vi "Strategy 5_Autotuning PID_With GUI_Modified for Testing - Backup.vi"() -> ()   [LabVIEW 2018]
doc: "This example demonstrates how to use the PID Design function to obtain PID parameters based on measured process."
uses:
  <vilib>/DAQmx/write.llb/DAQmx Write (Digital 1D Bool 1Chan 1Samp).vi
  <vilib>/DAQmx/read.llb/DAQmx Read (Analog 1D DBL NChan 1Samp).vi
  <vilib>/Instr/_visa.llb/VISA Configure Serial Port (Instr).vi
  <vilib>/DAQmx/create/channels.llb/DAQmx Create Channel (DO-Digital Output).vi
  <vilib>/DAQmx/miscellaneous.llb/DAQmx Fill In Error Info.vi
  <vilib>/addons/control/pid/pid.llb/PID Advanced (DBL).vi
  <vilib>/addons/control/pid/autopid.llb/PID Autotuning Design (Ziegler-Nichols).vi
  <vilib>/addons/control/pid/autopid.llb/PID Autotuning Design (Cohen-Coon).vi
  <vilib>/addons/control/pid/autopid.llb/PID Autotuning Design (Chien-Hrones-Reswick).vi
  <vilib>/addons/control/pid/autopid.llb/PID Autotuning Design (Internal Model Control).vi
  <vilib>/addons/control/pid/NI_PID_autopid.lvlib
  <vilib>/addons/control/pid/NI_PID_pid.lvlib
  <vilib>/ptbypt/NI_PtbyPt.lvlib
panel:
  in  "Set Point 1,5":dbl
  out "Real time Data 1,5":dbl[][](graph)
  in  "Set Point 3,4":dbl
  out "Real time Data 3,4":dbl[][](graph)
  in  "Set Point 2":dbl
  out "Real time Data 2":dbl[][](graph)
  in  "Set Point 7":dbl
  out "Real time Data 7":dbl[][](graph)
  in  "Set Point  6,8,9,10":dbl
  out "Real time Data 6,8,9,10":dbl[][](graph)
  in  "Set Point 11,12":dbl
  out "Real time Data -11,12":dbl[][](graph)
  out "error out":errorcluster {"code" format="%.0x"}
  in  "XYZAER":T1(array[cluster]) {"r" format="%1_6f"; "e" format="%1_6f"; "a" format="%1_6f"; "z" format="%1_6f"; "y" format="%1_6f"; "x" format="%1_6f"}
  out "Start Time Text":string
  out "Stop Time Text":string
  out "Elapsed Time Text":string
  out "HostFrameCount":u32
  out "Loop Iter":i32
  out "PnoData":bool
  in  "stop":bool
  out "?":bool
  in  "Muscle Control":T2(tab)=enum."M-11,12"
  out "Tuned PID gains 12":T3={"proportional gain (Kc)"=1.9838195929127882, "integral time (Ti, min)"=0.01995856284686879, "derivative time (Td, min)"=0.0} {"derivative time (Td, min)" format="%#.6g"; "integral time (Ti, min)" format="%#.6g"; "proportional gain (Kc)" format="%#.6g"}
  in  "Accept gain 12":bool
  in  "Control 12":T4(tab)
  in  "Ziegler-Nichols speed 12":u16(ring) items=["Fast", "Normal", "Slow"]
  in  "Tuning specifications 12":u16(ring) items=["Regulator - 0 %", "Regulator -  20%", "Servo - 0%", "Servo - 20%"]
  in  "Multiplicative factor 12":dbl(slide)=1.0 scale=0.01..100.0
  in  "Type of controller 12":u16(ring)=2 items=["P", "PI", "PID"]
  in  "Stop 12":bool
  in  "PID Gains 12":T3={"proportional gain (Kc)"=0.1625, "integral time (Ti, min)"=1.25, "derivative time (Td, min)"=0.0} {"derivative time (Td, min)" format="%#.6g"; "integral time (Ti, min)" format="%#.6g"; "proportional gain (Kc)" format="%#.6g"}
  in  "Autotune 12":bool
  in  "Reinitialize 12":bool
  in  "Excitation 12":dbl=0.5 format="%.2f"
  in  "Automatic 12":bool=TRUE
  in  "MV: 12":dbl(slide)=20.39115328927357 scale=-100.0..100.0
  out "PWM Output 12":bool
  in  "Median sample length 21":i32=100
  in  "INLET 1,5 ON/OFF 3":bool=TRUE
  out "Tuned PID gains 9":T3={"proportional gain (Kc)"=1.9838195929127882, "integral time (Ti, min)"=0.01995856284686879, "derivative time (Td, min)"=0.0} {"derivative time (Td, min)" format="%#.6g"; "integral time (Ti, min)" format="%#.6g"; "proportional gain (Kc)" format="%#.6g"}
  in  "Accept gain 9":bool
  in  "Type of controller 9":u16(ring)=2 items=["P", "PI", "PID"]
  in  "Excitation 9":dbl=0.5 format="%.2f"
  in  "Control 9":T4(tab)
  in  "Ziegler-Nichols speed 9":u16(ring) items=["Fast", "Normal", "Slow"]
  in  "Tuning specifications 9":u16(ring) items=["Regulator - 0 %", "Regulator -  20%", "Servo - 0%", "Servo - 20%"]
  in  "Multiplicative factor 9":dbl(slide)=1.0 scale=0.01..100.0
  in  "Stop 9":bool
  in  "PID Gains 9":T3={"proportional gain (Kc)"=0.1625, "integral time (Ti, min)"=1.25, "derivative time (Td, min)"=0.0} {"derivative time (Td, min)" format="%#.6g"; "integral time (Ti, min)" format="%#.6g"; "proportional gain (Kc)" format="%#.6g"}
  in  "Autotune 9":bool
  in  "Reinitialize 9":bool
  in  "Automatic 9":bool=TRUE
  in  "MV: 9":dbl(slide)=20.39115328927357 scale=-100.0..100.0
  out "PWM Output 9":bool
  in  "Median sample length 18":i32=100
  in  "INLET 3,4 ON/OFF 2":bool=TRUE
  out "Tuned PID gains 8":T3={"proportional gain (Kc)"=1.9838195929127882, "integral time (Ti, min)"=0.01995856284686879, "derivative time (Td, min)"=0.0} {"derivative time (Td, min)" format="%#.6g"; "integral time (Ti, min)" format="%#.6g"; "proportional gain (Kc)" format="%#.6g"}
  in  "Accept gain 8":bool
  in  "Control 8":T4(tab)
  in  "Ziegler-Nichols speed 8":u16(ring) items=["Fast", "Normal", "Slow"]
  in  "Tuning specifications 8":u16(ring) items=["Regulator - 0 %", "Regulator -  20%", "Servo - 0%", "Servo - 20%"]
  in  "Multiplicative factor 8":dbl(slide)=1.0 scale=0.01..100.0
  in  "Type of controller 8":u16(ring)=2 items=["P", "PI", "PID"]
  in  "Stop 8":bool
  in  "PID Gains 8":T3={"proportional gain (Kc)"=0.1625, "integral time (Ti, min)"=1.25, "derivative time (Td, min)"=0.0} {"derivative time (Td, min)" format="%#.6g"; "integral time (Ti, min)" format="%#.6g"; "proportional gain (Kc)" format="%#.6g"}
  in  "Autotune 8":bool
  in  "Reinitialize 8":bool
  in  "Excitation 8":dbl=0.5 format="%.2f"
  in  "Automatic 8":bool=TRUE
  in  "MV: 8":dbl(slide)=20.39115328927357 scale=-100.0..100.0
  out "PWM Output 8":bool
  in  "Median sample length 17":i32=100
  in  "INLET 2 ON/OFF 2":bool=TRUE
  out "Tuned PID gains 7":T3={"proportional gain (Kc)"=1.9838195929127882, "integral time (Ti, min)"=0.01995856284686879, "derivative time (Td, min)"=0.0} {"derivative time (Td, min)" format="%#.6g"; "integral time (Ti, min)" format="%#.6g"; "proportional gain (Kc)" format="%#.6g"}
  in  "Accept gain 7":bool
  in  "Control 7":T4(tab)
  in  "Ziegler-Nichols speed 7":u16(ring) items=["Fast", "Normal", "Slow"]
  in  "Tuning specifications 7":u16(ring) items=["Regulator - 0 %", "Regulator -  20%", "Servo - 0%", "Servo - 20%"]
  in  "Multiplicative factor 7":dbl(slide)=1.0 scale=0.01..100.0
  in  "Type of controller 7":u16(ring)=2 items=["P", "PI", "PID"]
  in  "Stop 7":bool
  in  "PID Gains 7":T3={"proportional gain (Kc)"=0.1625, "integral time (Ti, min)"=1.25, "derivative time (Td, min)"=0.0} {"derivative time (Td, min)" format="%#.6g"; "integral time (Ti, min)" format="%#.6g"; "proportional gain (Kc)" format="%#.6g"}
  in  "Autotune 7":bool
  in  "Reinitialize 7":bool
  in  "Excitation 7":dbl=0.5 format="%.2f"
  in  "Automatic 7":bool=TRUE
  in  "MV: 7":dbl(slide)=20.39115328927357 scale=-100.0..100.0
  out "PWM Output 7":bool
  in  "Median sample length 16":i32=100
  in  "INLET 7 ON/OFF 2":bool=TRUE
  out "Tuned PID gains 6":T3={"proportional gain (Kc)"=1.9838195929127882, "integral time (Ti, min)"=0.01995856284686879, "derivative time (Td, min)"=0.0} {"derivative time (Td, min)" format="%#.6g"; "integral time (Ti, min)" format="%#.6g"; "proportional gain (Kc)" format="%#.6g"}
  in  "Accept gain 6":bool
  in  "Control 6":T4(tab)
  in  "Ziegler-Nichols speed 6":u16(ring) items=["Fast", "Normal", "Slow"]
  in  "Tuning specifications 6":u16(ring) items=["Regulator - 0 %", "Regulator -  20%", "Servo - 0%", "Servo - 20%"]
  in  "Multiplicative factor 6":dbl(slide)=1.0 scale=0.01..100.0
  in  "Type of controller 6":u16(ring)=2 items=["P", "PI", "PID"]
  in  "Stop 6":bool
  in  "PID Gains 6":T3={"proportional gain (Kc)"=0.1625, "integral time (Ti, min)"=1.25, "derivative time (Td, min)"=0.0} {"derivative time (Td, min)" format="%#.6g"; "integral time (Ti, min)" format="%#.6g"; "proportional gain (Kc)" format="%#.6g"}
  in  "Autotune 6":bool
  in  "Reinitialize 6":bool
  in  "Excitation 6":dbl=0.5 format="%.2f"
  in  "Automatic 6":bool=TRUE
  in  "MV: 6":dbl(slide)=20.39115328927357 scale=-100.0..100.0
  out "PWM Output 6":bool
  in  "Median sample length 15":i32=100
  in  "INLET 6 ON/OFF 2":bool=TRUE
  in  "INLET":bool=TRUE
  out "PWM Output":bool
  in  "MV:":dbl(slide)=20.39115328927357 scale=-100.0..100.0
  in  "Median sample length":i32=100
  in  "Excitation":dbl=0.5 format="%.2f"
  in  "Type of controller":u16(ring)=2 items=["P", "PI", "PID"]
  in  "Control":T4(tab)
  in  "Ziegler-Nichols speed":u16(ring) items=["Fast", "Normal", "Slow"]
  in  "Tuning specifications":u16(ring) items=["Regulator - 0 %", "Regulator -  20%", "Servo - 0%", "Servo - 20%"]
  in  "Multiplicative factor":dbl(slide)=1.0 scale=0.01..100.0
  in  "Automatic":bool=TRUE
  in  "Reinitialize":bool
  in  "Accept gain":bool
  out "Tuned PID gains":T3={"proportional gain (Kc)"=1.9838195929127882, "integral time (Ti, min)"=0.01995856284686879, "derivative time (Td, min)"=0.0} {"derivative time (Td, min)" format="%#.6g"; "integral time (Ti, min)" format="%#.6g"; "proportional gain (Kc)" format="%#.6g"}
  in  "Autotune":bool
  in  "PID Gains":T3={"proportional gain (Kc)"=0.1625, "integral time (Ti, min)"=1.25, "derivative time (Td, min)"=0.0} {"derivative time (Td, min)" format="%#.6g"; "integral time (Ti, min)" format="%#.6g"; "proportional gain (Kc)" format="%#.6g"}
  in  "Stop":bool
  in  "M-11,12":i32=5
  in  "M-6,8,9,10":i32=5
  in  "M-7":i32=5
  in  "M-2":i32=5
  in  "M-3,4":i32=5
  in  "M-1,5":i32=5
  out "Stimulus operating point 12":dbl=20.314221540357543
  out "Response operating point 12":dbl=51.08345461694337
  out "Identified Plant Parameters 12":T5={"Plant Gain (K)"=1.7609511324977591, "Time Constant (T)"=1.9621978490901302, "Dead Time (L)"=0.22467425343567116}
  out "Control Output 12":dbl[](graph)
  out "Measurement 12":dbl[](graph)
  out "Stimulus operating point 9":dbl=20.314221540357543
  out "Response operating point 9":dbl=51.08345461694337
  out "Identified Plant Parameters 9":T5={"Plant Gain (K)"=1.7609511324977591, "Time Constant (T)"=1.9621978490901302, "Dead Time (L)"=0.22467425343567116}
  out "Control Output 9":dbl[](graph)
  out "Measurement 9":dbl[](graph)
  out "Identified Plant Parameters":T5={"Plant Gain (K)"=1.7609511324977591, "Time Constant (T)"=1.9621978490901302, "Dead Time (L)"=0.22467425343567116}
  out "Control Output":dbl[](graph)
  out "Measurement":dbl[](graph)
  out "Stimulus operating point":dbl=20.314221540357543
  out "Response operating point":dbl=51.08345461694337
  out "Stimulus operating point 6":dbl=20.314221540357543
  out "Response operating point 6":dbl=51.08345461694337
  out "Identified Plant Parameters 6":T5={"Plant Gain (K)"=1.7609511324977591, "Time Constant (T)"=1.9621978490901302, "Dead Time (L)"=0.22467425343567116}
  out "Control Output 6":dbl[](graph)
  out "Measurement 6":dbl[](graph)
  out "Stimulus operating point 7":dbl=20.314221540357543
  out "Response operating point 7":dbl=51.08345461694337
  out "Identified Plant Parameters 7":T5={"Plant Gain (K)"=1.7609511324977591, "Time Constant (T)"=1.9621978490901302, "Dead Time (L)"=0.22467425343567116}
  out "Control Output 7":dbl[](graph)
  out "Measurement 7":dbl[](graph)
  out "Stimulus operating point 8":dbl=20.314221540357543
  out "Response operating point 8":dbl=51.08345461694337
  out "Identified Plant Parameters 8":T5={"Plant Gain (K)"=1.7609511324977591, "Time Constant (T)"=1.9621978490901302, "Dead Time (L)"=0.22467425343567116}
  out "Control Output 8":dbl[](graph)
  out "Measurement 8":dbl[](graph)
  out "Connected":bool
  out "Running":bool
  out "Position Sensor Data":cluster{dbl, "x":sgl}[](graph)
  out "Sensor Raw Value 2":i32
  in  "COM Port-Sensor 2":refnum<visa-resource-name>="COM5"
  in  "upper/lower infle":enum32{"Page 1", "Page 2"}(tab)
  out "Force in Kilograms":dbl(graph)
  out "Force in Newtons":dbl(graph)
  in  "lower/upper infle":enum32{"Page 1", "Page 2"}(tab)
  out "Force in Newtons 2":dbl(graph)
  out "Force in Kilograms 2":dbl(graph)
  in  "COM Port-Sensor 1":refnum<visa-resource-name>="COM4"
  out "Sensor Raw Value":i32
  in  "Tab Control":T6(tab)
  in  "Instructions":string="Overview: This example demonstrates how to use the PID Autotuning Design to obtain PID parameters based on setpoint and process variable collected in another loop.\nInstructions:\n1. Run the VI and wait until the process variable (PV) reaches near setpoint (SP).\n2.  In the PID Autotuning Design section, select the type of algorithm, type of controller and excitation amplitude for the 'open loop step response'. Then, click Autotune to start the process. Select the Identified Plant Parameter tab and see the results from the identification.\n3.  When the tuned PID gains do not change anymore, the identification is done and you have the option to accept by clicking Accept gain, which will transfer the new gain to PID Gains.\n4. Click the Autotune button again to go back to the automatic control state. You can try different options and repeat this process.\n5. Click Stop to stop the VI.\n"
  # "Pressure Alarm"
  # "Force Sensor Data"
  # "Position Sensor Data"
  # "PID Controller"
  # "PID Autotuning Design"
  # "No additional parameters"
  # "PID Controller"
  # "PID Autotuning Design"
  # "No additional parameters"
  # "PID Controller"
  # "PID Autotuning Design"
  # "No additional parameters"
  # "PID Controller"
  # "PID Autotuning Design"
  # "No additional parameters"
  # "PID Controller"
  # "PID Autotuning Design"
  # "No additional parameters"
  # "Muscle Control"
  # "PID Controller"
  # "PID Autotuning Design"
  # "No additional parameters"
  # "Pressure Cut Off to trigger the alarm"
  # "M-11,12"
  # "M-3,4"
  # "M-1,5"
  # "M-6,8,9,10"
  # "M-7"
  # "M-2"
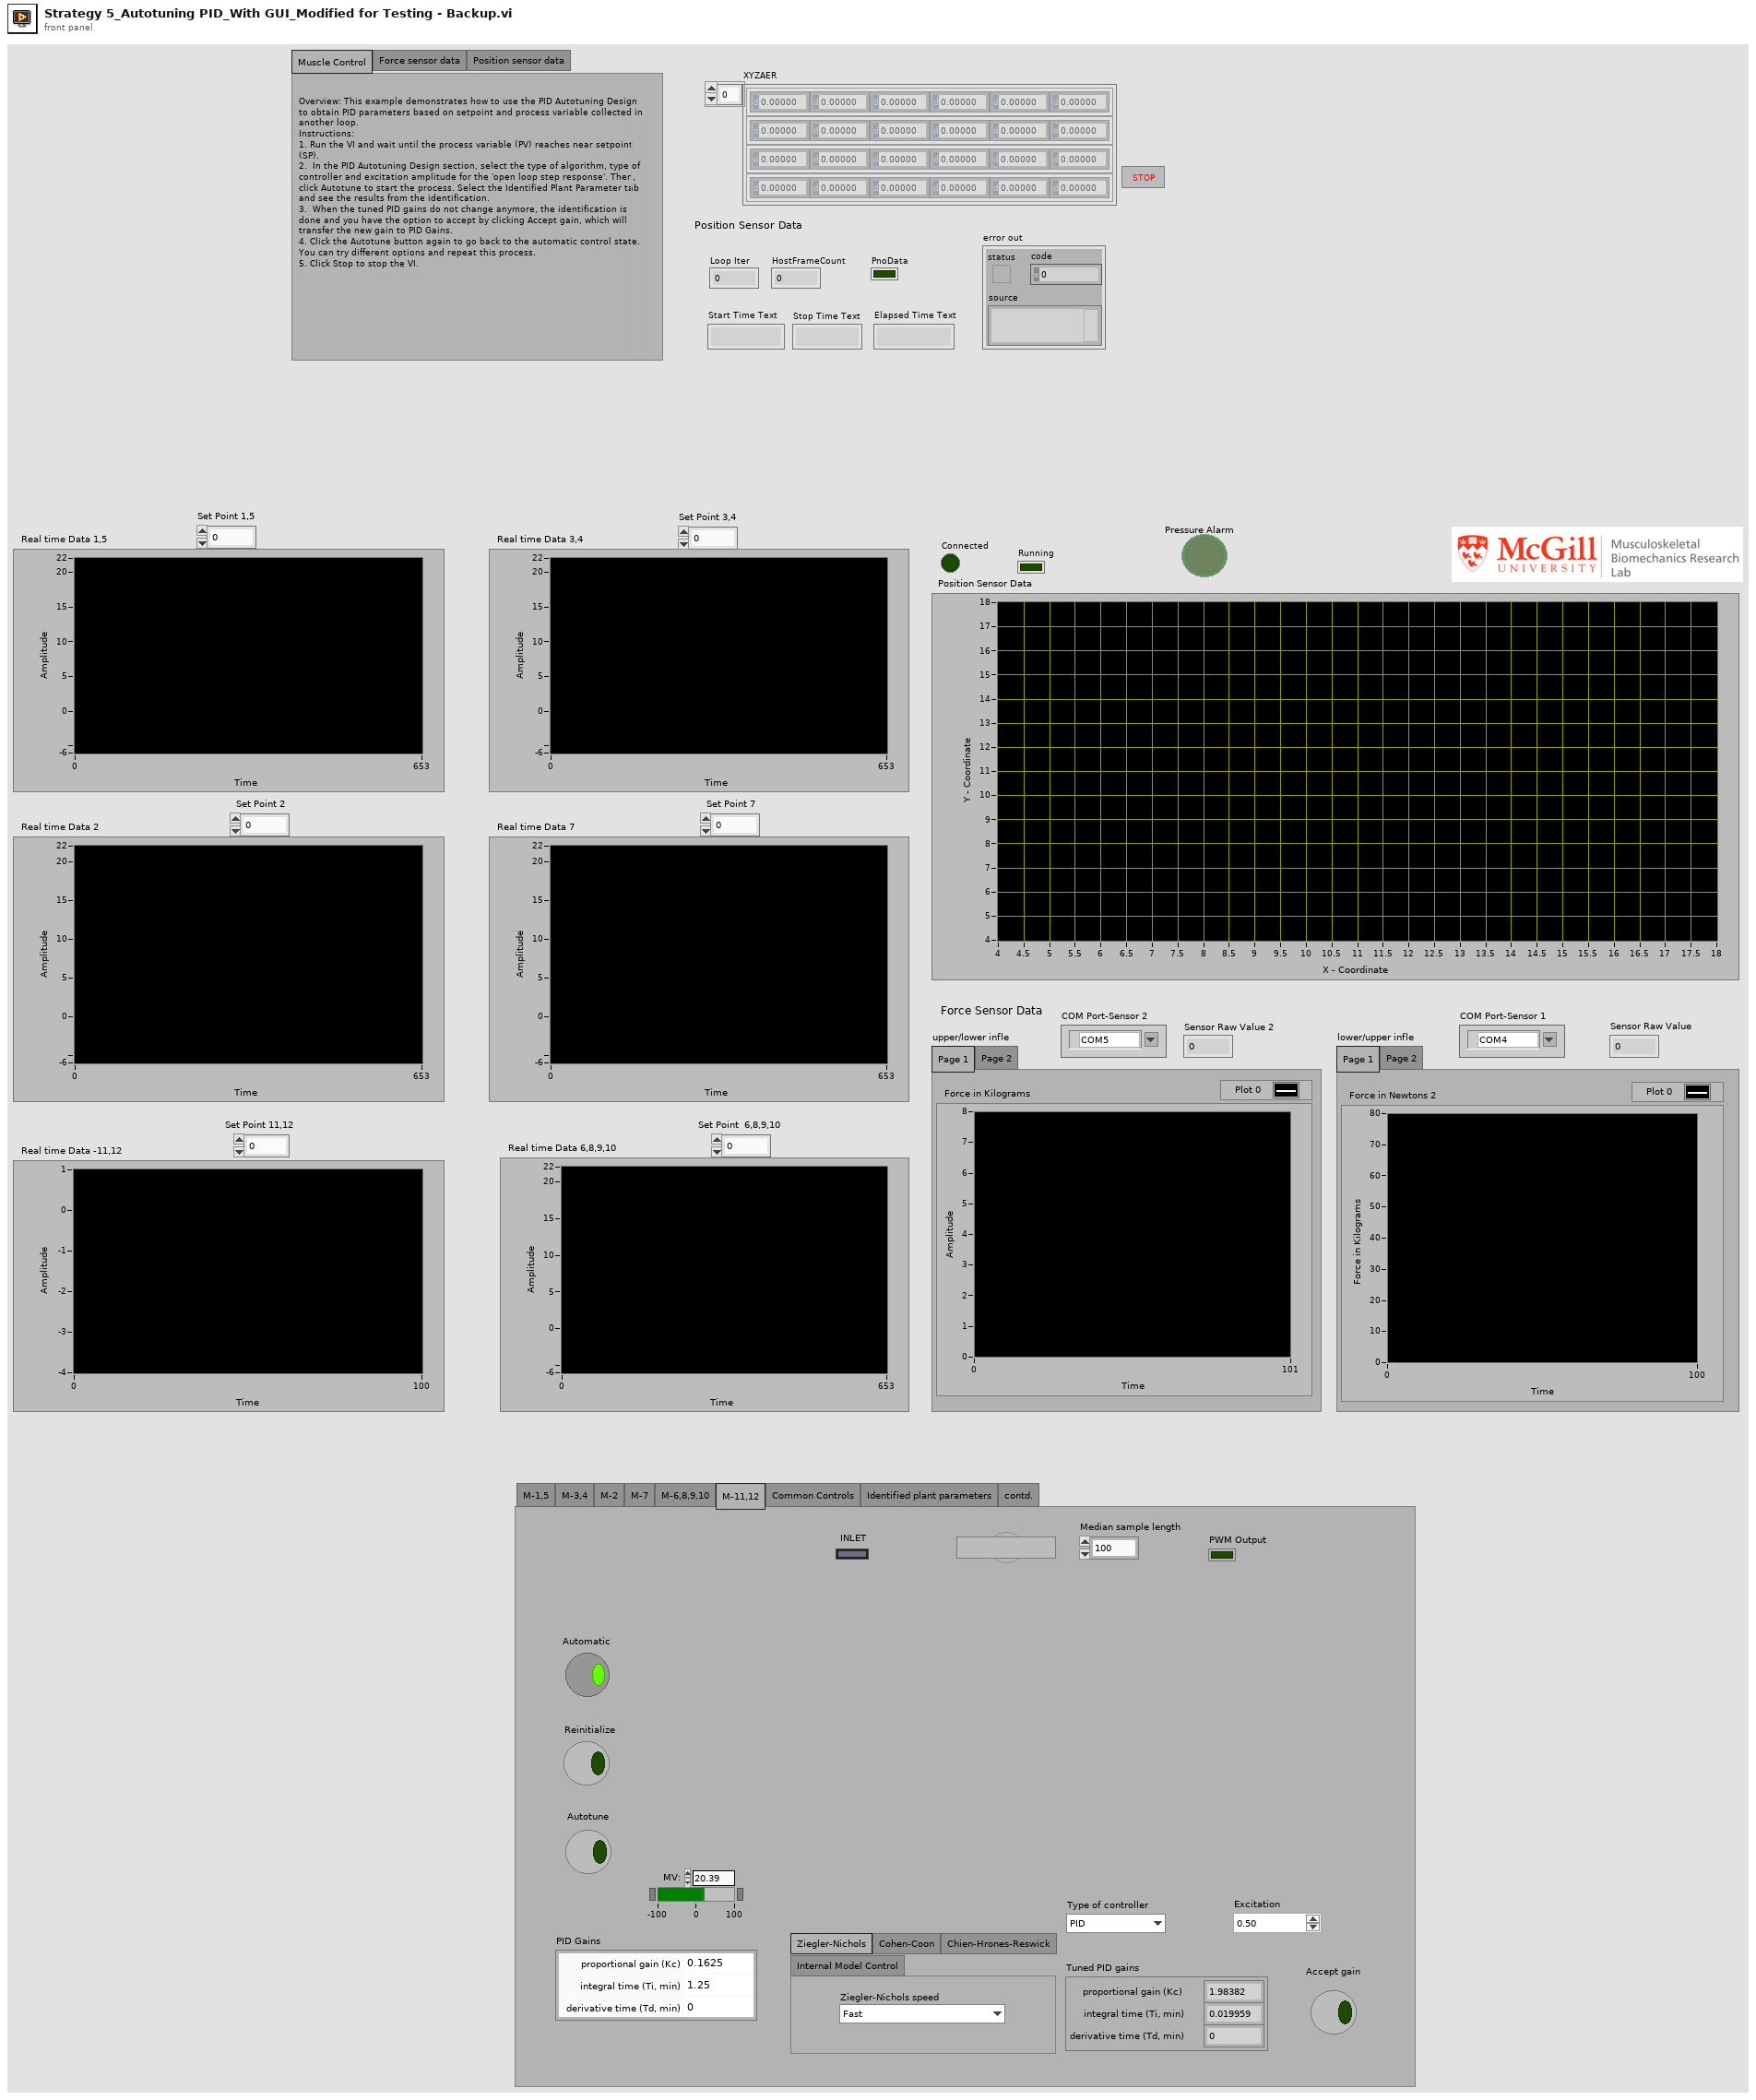
[diagram p1: front panel]
types:
  T1 = cluster{"x":sgl, "y":sgl, "z":sgl, "a":sgl, "e":sgl, "r":sgl}[]
  T2 = enum32{"M-1,5", "M-3,4", "M-2", "M-7", "M-6,8,9,10", "M-11,12", "Common Controls", "Identified plant parameters", "contd."}
  T3 = cluster{"proportional gain (Kc)":dbl, "integral time (Ti, min)":dbl, "derivative time (Td, min)":dbl}
  T4 = enum32{"Ziegler-Nichols", "Cohen-Coon", "Chien-Hrones-Reswick", "Internal Model Control"}
  T5 = cluster{"Plant Gain (K)":dbl, "Time Constant (T)":dbl, "Dead Time (L)":dbl}
  T6 = enum32{"Muscle Control", "Force sensor data", "Position sensor data"}
  T7 = cluster{"static gain":dbl, "lag (s)":dbl, "deadtime (s)":dbl, "load":dbl, "deadband":dbl, "sensor noise":dbl, "initial PV":dbl, "plant noise":dbl}
  T8 = cluster{"x":sgl, "y":sgl, "z":sgl, "a":sgl, "e":sgl, "r":sgl}
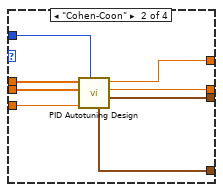
[diagram p2: hidden frame]
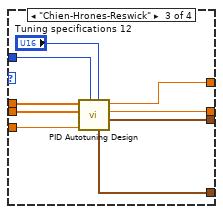
[diagram p3: hidden frame]
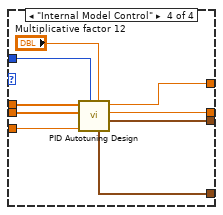
[diagram p4: hidden frame]
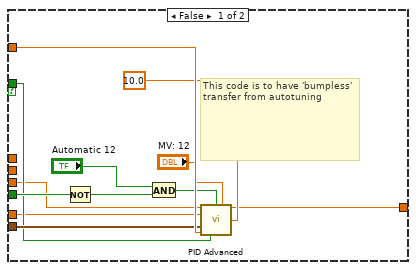
[diagram p6: hidden frame]
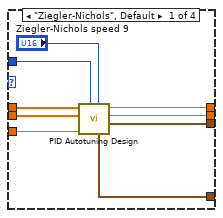
[diagram p7: hidden frame]
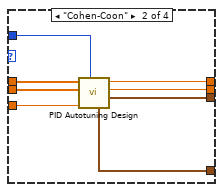
[diagram p8: hidden frame]
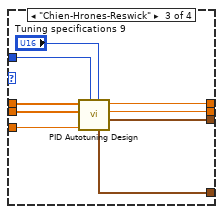
[diagram p9: hidden frame]
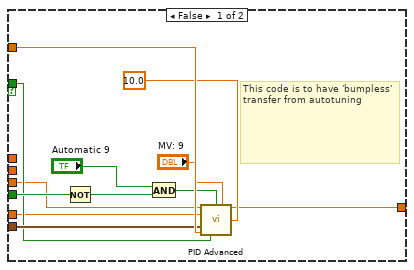
[diagram p11: hidden frame]
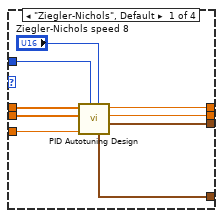
[diagram p12: hidden frame]
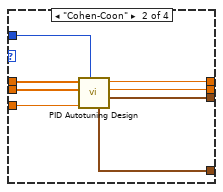
[diagram p13: hidden frame]
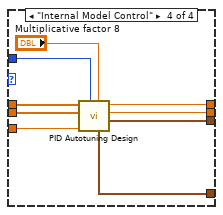
[diagram p14: hidden frame]
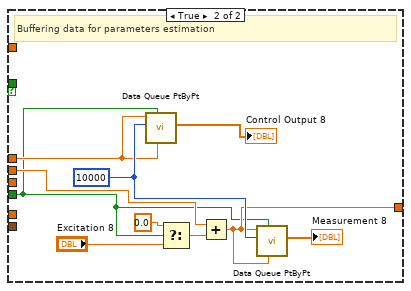
[diagram p16: hidden frame]
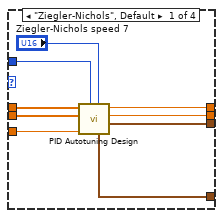
[diagram p17: hidden frame]
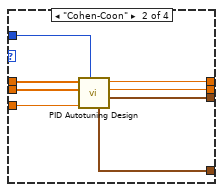
[diagram p18: hidden frame]
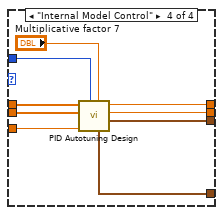
[diagram p19: hidden frame]
diagram:
  w19 = 0.0 ("output")
  w22 = FALSE ("Stop")
  w25 = 0.0 ("output")
  w28 = FALSE ("Stop")
  w31 = 0.0 ("output")
  w34 = FALSE ("Stop")
  w37 = 0.0 ("output")
  w40 = FALSE ("Stop")
  w43 = 0.0 ("output")
  w46 = FALSE ("Stop")
  w51 = 2400  # BufferFrameCount
  w85 = 0.0 ("output")
  w88 = FALSE ("Stop")
  # "Muscle-1,5 PID CONTROL LOOP (Auto Tuning)"
  # "Muscle-3,4 PID CONTROL LOOP (Auto Tuning)"
  # "Muscle-2 PID CONTROL LOOP (Auto Tuning)"
  # "Muscle-7 PID CONTROL LOOP (Auto Tuning)"
  # "Muscle-6,8,9,10 PID CONTROL LOOP (Auto Tuning)"
  # "Muscle-11,12 PID CONTROL LOOP (Auto Tuning)"
  # "FORCE SENSOR CONTROL LOOP"
  # "POSITION SENSOR CONTROL LOOP"
  # "Pressure Alarm"
  # "8. Close Tracker connection."
  # "3. Query Max num sensors supported by the tracker."
  # "4. Allocate raw buffer to hold 2400 frames of data."
  # "5. Start Continuous mode."
  # "7. Stop Continuous mode."
  # "6. Start the loop. Loop exits when Stop Button is hit."
  n1 = Obtain Queue(element data type=0.0) -> (queue out=w12:refnum<queue>)  [unwired: 4 in, 2 out]
  n2 = while {
    shift-left: 0.0 ("Plant Output") -> [w204]
    shift-right: [w199] -> _
    tunnel: w46 -> [_]
    shift-right: [w185] -> _
    shift-left: 0.01 -> [w183]
    shift-right: [w158] -> _
    shift-left: TRUE -> [w182]
    shift-right: [w160] -> _
    shift-left: w43 -> [w181]
    shift-right: [w184] -> _
    shift-left: w43 -> [w180]
    tunnel: [w155] -> w42
    tunnel: [w142] -> w2
    tunnel: w12 -> [w140]
    stop <- "Stop 6" stop-if-true
    w93 = 1 items=["one channel for each line", "one channel for all lines"] ("line grouping")
    w101 = 1 items=["one channel for each line", "one channel for all lines"] ("line grouping")
    w109 = 1 items=["one channel for each line", "one channel for all lines"] ("line grouping")
    w117 = 1 items=["one channel for each line", "one channel for all lines"] ("line grouping")
    w125 = 1 items=["one channel for each line", "one channel for all lines"] ("line grouping")
    w133 = 1 items=["one channel for each line", "one channel for all lines"] ("line grouping")
    w146 = 1 items=["one channel for each line", "one channel for all lines"] ("line grouping")
    w155 = 0.05 ("Sampling Time dt (s)")
    w163 = 1 items=["one channel for each line", "one channel for all lines"] ("line grouping")
    w171 = 0.5 ("x")
    w198 = T7 {"static gain"=2.5, "lag (s)"=2.5, "deadtime (s)"=0.01, "load"=0.0, "deadband"=0.0, "sensor noise"=0.0, "initial PV"=30.0, "plant noise"=0.0}  # Process parameters
    w200 = FALSE  # Integrator ?
    # "Inlet 11"
    # "Exhaust 10"
    # "Inlet 11"
    # "Exhaust 9"
    # "Inlet 11"
    # "Exhaust 8"
    # "C."
    # "Inlet 11"
    # "Exhaust 6"
    # "B."
    # "A."
    # "A.Output to PWM Logic \nB. Simulated Plant\nC. Draw Chart"
    # "Main PID Loop Control"
    n3 = Dequeue Element(queue=w140) -> (element=w141:dbl)  [unwired: 2 in, 3 out]
    n4 = Multiply(x=w155, y=1000.0) -> (x*y=w197:dbl)
    n5 = Not(x="Autotune 6") -> (.not. x?=w201:bool)
    n6 = feedback #1() -> (w206:bool)  [unwired: 1 in]
    n7 = feedback-in #1("Autotune 6") -> ()
    n8 = Wait Until Next ms Multiple(millisecond multiple=w197) -> ()  [unwired: 1 out]
    n9 = Exclusive Or(1:w206, 2:"Autotune 6") -> (0:w205:bool)
    n10 = feedback #2() -> (w203:dbl)  [unwired: 1 in]
    n11 = Multiply(x=w141, y=-1000.0) -> (x*y=w187:dbl)
    n12 = call <vilib>:"Median PtByPt.vi"("sample length"="Median sample length 15", "x"=w187) -> ("median"=w186:dbl)  [unwired: 2 in, 1 out]
    n13 = Square(x=w186) -> (x^2=w194:dbl)
    n14 = Multiply(x=w186, y=16.572) -> (x*y=w190:dbl)
    n15 = Multiply(x=w194, y=-0.06) -> (x*y=w191:dbl)
    n16 = Add(x=w190, y=w191) -> (x+y=w189:dbl)
    n17 = Add(x=-1011.3, y=w189) -> (x+y=w153:dbl)
    n18 = case shown="False" "Autotune 6" {
      tunnel: w155 -> [w221 _]
      tunnel: [w210 w226] -> w160
      tunnel: w204 -> [_ w225]
      tunnel: "PID Gains 6" -> [w220 _]
      tunnel: "Reinitialize 6" -> [w217 _]
      tunnel: w205 -> [w219 w224]
      tunnel: w203 -> [_ w228]
      tunnel: w153 -> [w213 _]
      tunnel: "Set Point  6,8,9,10" -> [w212 _]
      frame False {
        # "This code is to have 'bumpless' transfer from autotuning"
        n19 = Not(x=w219) -> (.not. x?=w216:bool)
        n20 = And(x="Automatic 6", y=w216) -> (x .and. y?=w218:bool)
        n21 = call-poly <vilib>:"PID Advanced.vi"("setpoint"=w212, "auto? (T)"=w218, "manual control"="MV: 6", "process variable"=w213, "alpha"=10.0, "PID gains"=w220, "dt (s)"=w221, "reinitialize? (F)"=w217) -> ("output"=w210:dbl)  [unwired: 6 in, 1 out]
      }
      frame True {
        w231 = 10000 ("sample length")
        # "Buffering data for parameters estimation"
        n22 = call <vilib>:"Data Queue PtByPt.vi"("initial queue element"=w225, "initialize"=w224, "sample length"=w231, "input data point"=w225) -> ("Current Queue"=→"Control Output 6":dbl[])  [unwired: 3 in, 4 out]
        n23 = Select(t=0.0, s=w224, f="Excitation 6") -> (s? t:f=w229:dbl)
        n24 = Add(x=w228, y=w229) -> (x+y=w226:dbl)
        n25 = call <vilib>:"Data Queue PtByPt.vi"("initial queue element"=w226, "initialize"=w224, "sample length"=w231, "input data point"=w226) -> ("Current Queue"=→"Measurement 6":dbl[])  [unwired: 3 in, 4 out]
      }
    }
    n26 = feedback-in #2(w160, w201) -> ()
    n27 = Greater?(x=w153, y="M-6,8,9,10") -> (0:w142:bool)
    n28 = Add(x=w183, y=w171) -> (x+y=w172:dbl)
    n29 = Subtract(x=w183, y=w171) -> (x-y=w170:dbl)
    n30 = Equal?(x=w181, y=w160) -> (x = y?=w178:bool)
    n31 = Greater?(x=w160, y=w181) -> (0:w177:bool)
    n32 = Select(t=w182, s=w178, f=w177) -> (s? t:f=w158:bool)
    "PWM Output 6" <- w158
    n33 = call "Plant System.vi"("Integrator ?"=w200, "Plant Input"=w160, "dt (s)"=w155, "process parameters"=w198) -> ("Plant Output"=w199:dbl)  [unwired: 11 in]
    n34 = Increment(x="Set Point  6,8,9,10") -> (x+1=w176:dbl)
    n35 = Decrement(x="Set Point  6,8,9,10") -> (x-1=w175:dbl)
    n36 = Select(t=w172, s=w158, f=w170) -> (s? t:f=w185:dbl)
    n37 = call-poly <vilib>:"DAQmx Create Virtual Channel.vi"("lines"=tag "cDAQ1Mod1/port0/line3", "line grouping"=w117) -> ("task out"=w119:refnum<k21>, "error out"=w118:errorcluster)  [unwired: 12 in]
    n38 = call-poly <vilib>:"DAQmx Create Virtual Channel.vi"("lines"=tag "cDAQ1Mod2/port0/line3", "line grouping"=w109) -> ("task out"=w111:refnum<k21>, "error out"=w110:errorcluster)  [unwired: 12 in]
    n39 = Select(t=w176, s=w158, f=w175) -> (s? t:f=w174:dbl)
    n40 = Not(x=w158) -> (.not. x?=w157:bool)
    n41 = call-poly <vilib>:"DAQmx Create Virtual Channel.vi"("lines"=tag "cDAQ1Mod1/port0/line4", "line grouping"=w163) -> ("task out"=w165:refnum<k21>, "error out"=w164:errorcluster)  [unwired: 12 in]
    n42 = call-poly <vilib>:"DAQmx Create Virtual Channel.vi"("lines"=tag "cDAQ1Mod2/port0/line4", "line grouping"=w146) -> ("task out"=w148:refnum<k21>, "error out"=w147:errorcluster)  [unwired: 12 in]
    n43 = Build Array(w153, "Set Point  6,8,9,10", w174) -> (w173:dbl[])
    n44 = Initialize Array("INLET 6 ON/OFF 2", 1 ("dimension size")) -> (w90:bool[])
    n45 = Initialize Array(w157, 1 ("dimension size")) -> (w91:bool[])
    n46 = local write "MV: 6"(w160) -> ()
    n47 = Add(x=w180, y=w183) -> (x+y=w184:dbl)
    n48 = Build Array(w173) -> (→"Real time Data 6,8,9,10":dbl[][])
    n49 = call-poly <vilib>:"DAQmx Write.vi"("task/channels in"=w119, "auto start"=TRUE, "data"=w91, "error in"=w118) -> ("task out"=w121:refnum<k21>, "error out"=w122:errorcluster)  [unwired: 9 in, 1 out]
    n50 = call-poly <vilib>:"DAQmx Write.vi"("task/channels in"=w111, "auto start"=TRUE, "data"=w90, "error in"=w110) -> ("task out"=w113:refnum<k21>, "error out"=w114:errorcluster)  [unwired: 9 in, 1 out]
    n51 = call-poly <vilib>:"DAQmx Write.vi"("task/channels in"=w165, "auto start"=TRUE, "data"=w91, "error in"=w164) -> ("task out"=w167:refnum<k21>, "error out"=w168:errorcluster)  [unwired: 9 in, 1 out]
    n52 = call-poly <vilib>:"DAQmx Write.vi"("task/channels in"=w148, "auto start"=TRUE, "data"=w90, "error in"=w147) -> ("task out"=w150:refnum<k21>, "error out"=w151:errorcluster)  [unwired: 9 in, 1 out]
    n53 = call <vilib>:"DAQmx Clear Task.vi"("task in"=w121, "error in"=w122) -> ("error out"=w116:errorcluster)  [unwired: 13 in]
    n54 = call <vilib>:"DAQmx Clear Task.vi"("task in"=w113, "error in"=w114) -> ("error out"=w108:errorcluster)  [unwired: 13 in]
    n55 = call <vilib>:"DAQmx Clear Task.vi"("task in"=w167, "error in"=w168) -> ("error out"=w162:errorcluster)  [unwired: 13 in]
    n56 = call <vilib>:"DAQmx Clear Task.vi"("task in"=w150, "error in"=w151) -> ("error out"=w145:errorcluster)  [unwired: 13 in]
    n57 = call <vilib>:"Simple Error Handler.vi"("error in (no error)"=w116) -> ()  [unwired: 4 in, 5 out]
    n58 = call <vilib>:"Simple Error Handler.vi"("error in (no error)"=w108) -> ()  [unwired: 4 in, 5 out]
    n59 = call <vilib>:"Simple Error Handler.vi"("error in (no error)"=w162) -> ()  [unwired: 4 in, 5 out]
    n60 = call <vilib>:"Simple Error Handler.vi"("error in (no error)"=w145) -> ()  [unwired: 4 in, 5 out]
    n61 = call-poly <vilib>:"DAQmx Create Virtual Channel.vi"("lines"=tag "cDAQ1Mod8/port0/line6", "line grouping"=w101) -> ("task out"=w103:refnum<k21>, "error out"=w102:errorcluster)  [unwired: 12 in]
    n62 = call-poly <vilib>:"DAQmx Create Virtual Channel.vi"("lines"=tag "cDAQ1Mod7/port0/line5", "line grouping"=w93) -> ("task out"=w95:refnum<k21>, "error out"=w94:errorcluster)  [unwired: 12 in]
    n63 = call-poly <vilib>:"DAQmx Create Virtual Channel.vi"("lines"=tag "cDAQ1Mod8/port0/line3", "line grouping"=w133) -> ("task out"=w135:refnum<k21>, "error out"=w134:errorcluster)  [unwired: 12 in]
    n64 = call-poly <vilib>:"DAQmx Create Virtual Channel.vi"("lines"=tag "cDAQ1Mod7/port0/line2", "line grouping"=w125) -> ("task out"=w127:refnum<k21>, "error out"=w126:errorcluster)  [unwired: 12 in]
    n65 = call-poly <vilib>:"DAQmx Write.vi"("task/channels in"=w103, "auto start"=TRUE, "data"=w91, "error in"=w102) -> ("task out"=w105:refnum<k21>, "error out"=w106:errorcluster)  [unwired: 9 in, 1 out]
    n66 = call-poly <vilib>:"DAQmx Write.vi"("task/channels in"=w95, "auto start"=TRUE, "data"=w90, "error in"=w94) -> ("task out"=w97:refnum<k21>, "error out"=w98:errorcluster)  [unwired: 9 in, 1 out]
    n67 = call-poly <vilib>:"DAQmx Write.vi"("task/channels in"=w135, "auto start"=TRUE, "data"=w91, "error in"=w134) -> ("task out"=w137:refnum<k21>, "error out"=w138:errorcluster)  [unwired: 9 in, 1 out]
    n68 = call-poly <vilib>:"DAQmx Write.vi"("task/channels in"=w127, "auto start"=TRUE, "data"=w90, "error in"=w126) -> ("task out"=w129:refnum<k21>, "error out"=w130:errorcluster)  [unwired: 9 in, 1 out]
    n69 = call <vilib>:"DAQmx Clear Task.vi"("task in"=w105, "error in"=w106) -> ("error out"=w100:errorcluster)  [unwired: 13 in]
    n70 = call <vilib>:"DAQmx Clear Task.vi"("task in"=w97, "error in"=w98) -> ("error out"=w92:errorcluster)  [unwired: 13 in]
    n71 = call <vilib>:"DAQmx Clear Task.vi"("task in"=w137, "error in"=w138) -> ("error out"=w132:errorcluster)  [unwired: 13 in]
    n72 = call <vilib>:"DAQmx Clear Task.vi"("task in"=w129, "error in"=w130) -> ("error out"=w124:errorcluster)  [unwired: 13 in]
    n73 = call <vilib>:"Simple Error Handler.vi"("error in (no error)"=w100) -> ()  [unwired: 4 in, 5 out]
    n74 = call <vilib>:"Simple Error Handler.vi"("error in (no error)"=w92) -> ()  [unwired: 4 in, 5 out]
    n75 = call <vilib>:"Simple Error Handler.vi"("error in (no error)"=w132) -> ()  [unwired: 4 in, 5 out]
    n76 = call <vilib>:"Simple Error Handler.vi"("error in (no error)"=w124) -> ()  [unwired: 4 in, 5 out]
  }
  n77 = local write "Stop 6"(w46) -> ()
  n78 = while {
    tunnel: w46 -> [_]
    tunnel: w42 -> [w235]
    stop <- w245 stop-if-true
    # "If dT and deadtime have similar values, the identification could evaluate deadtime as zero and this generates proportional gain equal to Inf. This code avoid gain changes in this situations."
    # "Autotuning Loop"
    n79 = local read "Control Output 6"() -> (w247:dbl[])
    n80 = local read "Measurement 6"() -> (w246:dbl[])
    n81 = case shown="\"Chien-Hrones-Reswick\"" "Control 6" {
      tunnel: w247 -> [w256 w264 w273 w282]
      tunnel: w246 -> [w255 w263 w272 w281]
      tunnel: [w254 w262 w271 w280] -> w234
      tunnel: [w253 w261 w270 w279] -> w233
      tunnel: w235 -> [w252 w260 w269 w278]
      tunnel: [w251 w259 w268 w277] -> w232
      tunnel: [w250 w258 w267 w276] -> w237
      tunnel: "Type of controller 6" -> [w249 w257 w266 w275]
      frame "Ziegler-Nichols", Default {
        n82 = call-poly <vilib>:"PID Autotuning Design.vi"("Ziegler-Nichols Speed"="Ziegler-Nichols speed 6", "Type of Controller"=w249, "dt (s)"=w252, "Response signal"=w255, "Stimulus signal"=w256) -> ("PID gains"=w250:T3, "response operating point"=w253:dbl, "stimulus operating point"=w254:dbl, "Plant Parameters"=w251:T5)  [unwired: 3 in]
      }
      frame "Cohen-Coon" {
        n83 = call-poly <vilib>:"PID Autotuning Design.vi"("Type of Controller"=w257, "dt (s)"=w260, "Response signal"=w263, "Stimulus signal"=w264) -> ("PID gains"=w258:T3, "response offset"=w261:dbl, "stimulus offset"=w262:dbl, "Plant Parameters"=w259:T5)  [unwired: 4 in]
      }
      frame "Chien-Hrones-Reswick" {
        n84 = call-poly <vilib>:"PID Autotuning Design.vi"("Tuning specifications"="Tuning specifications 6", "Type of Controller"=w266, "dt (s)"=w269, "Response signal"=w272, "Stimulus signal"=w273) -> ("PID gains"=w267:T3, "response offset"=w270:dbl, "stimulus offset"=w271:dbl, "Plant Parameters"=w268:T5)  [unwired: 3 in]
      }
      frame "Internal Model Control" {
        n85 = call-poly <vilib>:"PID Autotuning Design.vi"("Desired Time Constant (tau_c)"="Multiplicative factor 6", "Type of Controller"=w275, "dt (s)"=w278, "Response signal"=w281, "Stimulus signal"=w282) -> ("PID gains"=w276:T3, "response offset"=w279:dbl, "stimulus offset"=w280:dbl, "Plant Parameters"=w277:T5)  [unwired: 3 in]
      }
    }
    "Stimulus operating point 6" <- w234
    "Response operating point 6" <- w233
    "Identified Plant Parameters 6" <- w232
    n86 = Unbundle(w237) -> ("proportional gain (Kc)"=w240:dbl)  [unwired: 2 out]
    n87 = Equal?(x=w240, y=inf) -> (x = y?=w239:bool)
    n88 = feedback #3() -> (w238:T3)  [unwired: 1 in]
    n89 = Select(t=w238, s=w239, f=w237) -> (s? t:f=w236:T3)
    "Tuned PID gains 6" <- w236
    n90 = feedback-in #3(w236) -> ()
    n91 = case shown="True" "Accept gain 6" {
      tunnel: w236 -> [_ w283]
      frame False {
      }
      frame True {
        n92 = local write "PID Gains 6"(w283) -> ()
      }
    }
    n93 = local read "Stop 6"() -> (w245:bool)
  }
  n94 = local write "Stop"(w88) -> ()
  n95 = call-poly "VISA Configure Serial Port"("VISA resource name"="COM Port-Sensor 1") -> ("VISA resource name out"=w79:refnum<visa-resource-name>, "error out"=w78:errorcluster)  [unwired: 9 in, 4 out]
  n96 = call-poly "VISA Configure Serial Port"("VISA resource name"="COM Port-Sensor 2") -> ("VISA resource name out"=w74:refnum<visa-resource-name>, "error out"=w73:errorcluster)  [unwired: 9 in, 4 out]
  n97 = while {
    shift-right: [w291] -> w80
    shift-left: w79 -> [w287]
    tunnel: w78 -> [w286]
    tunnel: [w288] -> w81
    stop <- w289 stop-if-true
    # "Serial Read Loop"
    n98 = case shown="True" TRUE {
      tunnel: [w303 w307] -> w291
      tunnel: w287 -> [w305 w307]
      tunnel: [w302 w306] -> w288
      tunnel: w286 -> [w304 w306]
      frame True {
        n99 = VISA Read(VISA resource name=w305, byte count=u32 1000, error in (no error)=w304) -> (VISA resource name out=w303:refnum<visa-resource-name>, read buffer=w300:string, error out=w302:errorcluster)  [unwired: 1 out]
        n100 = Decimal String To Number(string=w300) -> (number=w298:i32)  [unwired: 2 in, 1 out]
        "Sensor Raw Value" <- w298
        n101 = call <vilib>:"Median PtByPt.vi"("sample length"=20, "x"=w298) -> ("median"=w296:dbl)  [unwired: 2 in, 1 out]
        n102 = To Double Precision Float(number=w296) -> (double precision float=w292:dbl)
        n103 = Multiply(x=w292, y=0.0292) -> (x*y=w295:dbl)
        "Force in Kilograms 2" <- w295
        n104 = Multiply(x=w295, y=9.81) -> (x*y=→"Force in Newtons 2":dbl)
      }
      frame False {
      }
    }
    n105 = Wait (ms)(milliseconds to wait=u32 5) -> ()  [unwired: 1 out]
    n106 = Or(x=w288, y=FALSE) -> (x .or. y?=w289:bool)
  }
  n107 = while {
    shift-right: [w315] -> w48
    shift-left: w74 -> [w311]
    tunnel: w73 -> [w310]
    tunnel: [w312] -> w75
    stop <- w313 stop-if-true
    # "Serial Read Loop"
    n108 = case shown="True" TRUE {
      tunnel: [w327 w331] -> w315
      tunnel: w311 -> [w329 w331]
      tunnel: [w326 w330] -> w312
      tunnel: w310 -> [w328 w330]
      frame True {
        n109 = VISA Read(VISA resource name=w329, byte count=u32 1000, error in (no error)=w328) -> (VISA resource name out=w327:refnum<visa-resource-name>, read buffer=w324:string, error out=w326:errorcluster)  [unwired: 1 out]
        n110 = Decimal String To Number(string=w324) -> (number=w320:i32)  [unwired: 2 in, 1 out]
        "Sensor Raw Value 2" <- w320
        n111 = call <vilib>:"Median PtByPt.vi"("sample length"=20, "x"=w320) -> ("median"=w321:dbl)  [unwired: 2 in, 1 out]
        n112 = To Double Precision Float(number=w321) -> (double precision float=w317:dbl)
        n113 = Multiply(x=w317, y=0.0238) -> (x*y=w316:dbl)
        "Force in Kilograms" <- w316
        n114 = Multiply(x=w316, y=9.81) -> (x*y=→"Force in Newtons":dbl)
      }
      frame False {
      }
    }
    n115 = Or(x=w312, y=FALSE) -> (x .or. y?=w313:bool)
    n116 = Wait (ms)(milliseconds to wait=u32 5) -> ()  [unwired: 1 out]
  }
  n117 = VISA Close(VISA resource name=w80, error in (no error)=w81) -> (error out=w82:errorcluster)
  n118 = call <vilib>:"Simple Error Handler.vi"("error in (no error)"=w82) -> ()  [unwired: 1 in, 8 out]
  n119 = VISA Close(VISA resource name=w48, error in (no error)=w75) -> (error out=w76:errorcluster)
  n120 = call <vilib>:"Simple Error Handler.vi"("error in (no error)"=w76) -> ()  [unwired: 1 in, 8 out]
  n121 = stacked-sequence {
    tunnel: [_ w337] -> w55
    tunnel: [_ w336] -> w54
    frame #0 {
      w332 = 0
      w333 = FALSE
      w334 = ""
      # "Initialize Indicators"
      "Connected" <- w333
      "Start Time Text" <- w334
      "Stop Time Text" <- w334
      "Elapsed Time Text" <- w334
      "HostFrameCount" <- w332
      "Running" <- w333
      "Loop Iter" <- w332
      "PnoData" <- w333
    }
    frame #1 {
      # "Connect To Tracker"
      # "2. Initialize Tracker Connection"
      n122 = call <instrlib>:"PDI initialize.vi"() -> ("error out"=w336:errorcluster, "Connected"=w335:bool, "pDev"=w337:u32)  [unwired: 1 in, 4 out]
      n123 = local write "Connected"(w335) -> ()
    }
  }
  n124 = while {
    stop <- FALSE stop-if-true
    # "TRACKER 4"
    # "TRACKER 3"
    # "TRACKER 2"
    # "TRACKER 1"
    n125 = Index Array(array="XYZAER", index #1=0 ("index"), index #2=1 ("index"), index #3=2 ("index"), index #4=3 ("index")) -> (element #1=w362:T8, element #2=w361:T8, element #3=w360:T8, element #4=w359:T8)
    n126 = Unbundle By Name(w362) -> ("x"=w349:sgl, "y"=w348:sgl)  [unwired: 1 out]
    n127 = Unbundle By Name(w361) -> ("x"=w346:sgl, "y"=w345:sgl)  [unwired: 1 out]
    n128 = Multiply(x=w348, y=sgl -1.0) -> (x*y=w347:sgl)
    n129 = Multiply(x=w345, y=-1.0) -> (x*y=w344:dbl)
    n130 = Bundle(w344, "x"=w346) -> (w357:cluster{dbl, "x":sgl})  [unwired: 1 in]
    n131 = Bundle(w347, "x"=w349) -> (w358:cluster{sgl, "x":sgl})  [unwired: 1 in]
    n132 = Unbundle By Name(w360) -> ("x"=w343:sgl, "y"=w342:sgl)  [unwired: 1 out]
    n133 = Unbundle By Name(w359) -> ("x"=w340:sgl, "y"=w339:sgl)  [unwired: 1 out]
    n134 = Multiply(x=w342, y=-1.0) -> (x*y=w341:dbl)
    n135 = Multiply(x=w339, y=-1.0) -> (x*y=w338:dbl)
    n136 = Bundle(w341, "x"=w343) -> (w356:cluster{dbl, "x":sgl})  [unwired: 1 in]
    n137 = Bundle(w338, "x"=w340) -> (w355:cluster{dbl, "x":sgl})  [unwired: 1 in]
    n138 = Build Array(w358, w357, w356, w355) -> (→"Position Sensor Data":cluster{dbl, "x":sgl}[])
  }
  n139 = call <instrlib>:"PDI util stationcount.vi"("error in (no error)"=w54, "pDev"=w55) -> ("error out"=w53:errorcluster, "dup pDev"=w52:u32, "MaxCount"=w50:i32)  [unwired: 7 out]
  n140 = call <instrlib>:"PDI config setbuffer.vi"("error in (no error)"=w53, "Max sensors"=w50, "FrameCount"=w51, "pDev"=w52) -> ("error out"=w62:errorcluster, "dup pDev"=w63:u32)  [unwired: 6 out]
  n141 = flat-sequence {
    tunnel: w68 -> [_]
    tunnel: [w369] -> w64
    frame #0 {
      # "Get Start Time"
      n142 = Get Date/Time In Seconds() -> (seconds since 1Jan1904=w370:timestamp)
      n143 = Format Date/Time String(seconds (now)=w370) -> (date/time string=w371:string)  [unwired: 2 out]
      n144 = local write "Start Time Text"(w371) -> ()
      n145 = To Double Precision Float(number=w370) -> (double precision float=w369:dbl)
    }
  }
  n146 = call <instrlib>:"PDI action startcont.vi"("error in (no error)"=w62, "pDev"=w63) -> ("error out"=w69:errorcluster, "Running"=w61:bool, "dup pDev"=w68:u32)  [unwired: 7 out]
  n147 = control-ref of="HostFrameCount"() -> (w59:refnum<vi>)
  n148 = local write "Running"(w61) -> ()
  n149 = Obtain Queue(element data type=0.0) -> (queue out=w8:refnum<queue>)  [unwired: 4 in, 2 out]
  n150 = while {
    shift-left: 0.0 ("Plant Output") -> [w454]
    shift-right: [w449] -> _
    tunnel: w28 -> [_]
    shift-right: [w435] -> _
    shift-left: 0.01 -> [w433]
    shift-right: [w408] -> _
    shift-left: TRUE -> [w432]
    shift-right: [w410] -> _
    shift-left: w25 -> [w431]
    shift-right: [w434] -> _
    shift-left: w25 -> [w430]
    tunnel: [w405] -> w24
    tunnel: [w393] -> w16
    tunnel: w8 -> [w391]
    stop <- "Stop 9" stop-if-true
    w376 = 1 items=["one channel for each line", "one channel for all lines"] ("line grouping")
    w384 = 1 items=["one channel for each line", "one channel for all lines"] ("line grouping")
    w396 = 1 items=["one channel for each line", "one channel for all lines"] ("line grouping")
    w405 = 0.05 ("Sampling Time dt (s)")
    w413 = 1 items=["one channel for each line", "one channel for all lines"] ("line grouping")
    w421 = 0.5 ("x")
    w448 = T7 {"static gain"=2.5, "lag (s)"=2.5, "deadtime (s)"=0.01, "load"=0.0, "deadband"=0.0, "sensor noise"=0.0, "initial PV"=30.0, "plant noise"=0.0}  # Process parameters
    w450 = FALSE  # Integrator ?
    # "Inlet 11"
    # "Exhaust 3"
    # "C."
    # "Inlet 11"
    # "Exhaust 4"
    # "B."
    # "A."
    # "A.Output to PWM Logic \nB. Simulated Plant\nC. Draw Chart"
    # "Main PID Loop Control"
    n151 = Dequeue Element(queue=w391) -> (element=w392:dbl)  [unwired: 2 in, 3 out]
    n152 = Multiply(x=w405, y=1000.0) -> (x*y=w447:dbl)
    n153 = Not(x="Autotune 9") -> (.not. x?=w451:bool)
    n154 = feedback #4() -> (w456:bool)  [unwired: 1 in]
    n155 = feedback-in #4("Autotune 9") -> ()
    n156 = Wait Until Next ms Multiple(millisecond multiple=w447) -> ()  [unwired: 1 out]
    n157 = Exclusive Or(1:w456, 2:"Autotune 9") -> (0:w455:bool)
    n158 = feedback #5() -> (w453:dbl)  [unwired: 1 in]
    n159 = Multiply(x=w392, y=-1000.0) -> (x*y=w437:dbl)
    n160 = call <vilib>:"Median PtByPt.vi"("sample length"="Median sample length 18", "x"=w437) -> ("median"=w436:dbl)  [unwired: 2 in, 1 out]
    n161 = Square(x=w436) -> (x^2=w444:dbl)
    n162 = Multiply(x=w436, y=0.1121) -> (x*y=w440:dbl)
    n163 = Multiply(x=w444, y=0.0243) -> (x*y=w441:dbl)
    n164 = Add(x=w440, y=w441) -> (x+y=w439:dbl)
    n165 = Add(x=-235.77, y=w439) -> (x+y=w403:dbl)
    n166 = case shown="True" "Autotune 9" {
      tunnel: w405 -> [w471 _]
      tunnel: [w460 w476] -> w410
      tunnel: w454 -> [_ w475]
      tunnel: "PID Gains 9" -> [w470 _]
      tunnel: "Reinitialize 9" -> [w467 _]
      tunnel: w455 -> [w469 w474]
      tunnel: w453 -> [_ w478]
      tunnel: w403 -> [w463 _]
      tunnel: "Set Point 3,4" -> [w462 _]
      frame False {
        # "This code is to have 'bumpless' transfer from autotuning"
        n167 = Not(x=w469) -> (.not. x?=w466:bool)
        n168 = And(x="Automatic 9", y=w466) -> (x .and. y?=w468:bool)
        n169 = call-poly <vilib>:"PID Advanced.vi"("setpoint"=w462, "auto? (T)"=w468, "manual control"="MV: 9", "process variable"=w463, "alpha"=10.0, "PID gains"=w470, "dt (s)"=w471, "reinitialize? (F)"=w467) -> ("output"=w460:dbl)  [unwired: 6 in, 1 out]
      }
      frame True {
        w481 = 10000 ("sample length")
        # "Buffering data for parameters estimation"
        n170 = call <vilib>:"Data Queue PtByPt.vi"("initial queue element"=w475, "initialize"=w474, "sample length"=w481, "input data point"=w475) -> ("Current Queue"=→"Control Output 9":dbl[])  [unwired: 3 in, 4 out]
        n171 = Select(t=0.0, s=w474, f="Excitation 9") -> (s? t:f=w479:dbl)
        n172 = Add(x=w478, y=w479) -> (x+y=w476:dbl)
        n173 = call <vilib>:"Data Queue PtByPt.vi"("initial queue element"=w476, "initialize"=w474, "sample length"=w481, "input data point"=w476) -> ("Current Queue"=→"Measurement 9":dbl[])  [unwired: 3 in, 4 out]
      }
    }
    n174 = feedback-in #5(w410, w451) -> ()
    n175 = Greater?(x=w403, y="M-3,4") -> (0:w393:bool)
    n176 = Add(x=w433, y=w421) -> (x+y=w422:dbl)
    n177 = Subtract(x=w433, y=w421) -> (x-y=w420:dbl)
    n178 = Equal?(x=w431, y=w410) -> (x = y?=w428:bool)
    n179 = Greater?(x=w410, y=w431) -> (0:w427:bool)
    n180 = Select(t=w432, s=w428, f=w427) -> (s? t:f=w408:bool)
    "PWM Output 9" <- w408
    n181 = call "Plant System.vi"("Integrator ?"=w450, "Plant Input"=w410, "dt (s)"=w405, "process parameters"=w448) -> ("Plant Output"=w449:dbl)  [unwired: 11 in]
    n182 = Increment(x="Set Point 3,4") -> (x+1=w426:dbl)
    n183 = Decrement(x="Set Point 3,4") -> (x-1=w425:dbl)
    n184 = Select(t=w422, s=w408, f=w420) -> (s? t:f=w435:dbl)
    n185 = Select(t=w426, s=w408, f=w425) -> (s? t:f=w424:dbl)
    n186 = Not(x=w408) -> (.not. x?=w407:bool)
    n187 = call-poly <vilib>:"DAQmx Create Virtual Channel.vi"("lines"=tag "cDAQ1Mod8/port0/line5", "line grouping"=w413) -> ("task out"=w415:refnum<k21>, "error out"=w414:errorcluster)  [unwired: 12 in]
    n188 = call-poly <vilib>:"DAQmx Create Virtual Channel.vi"("lines"=tag "cDAQ1Mod7/port0/line4", "line grouping"=w396) -> ("task out"=w398:refnum<k21>, "error out"=w397:errorcluster)  [unwired: 12 in]
    n189 = Build Array(w403, "Set Point 3,4", w424) -> (w423:dbl[])
    n190 = Initialize Array("INLET 3,4 ON/OFF 2", 1 ("dimension size")) -> (w372:bool[])
    n191 = Initialize Array(w407, 1 ("dimension size")) -> (w374:bool[])
    n192 = local write "MV: 9"(w410) -> ()
    n193 = Add(x=w430, y=w433) -> (x+y=w434:dbl)
    n194 = Build Array(w423) -> (→"Real time Data 3,4":dbl[][])
    n195 = call-poly <vilib>:"DAQmx Write.vi"("task/channels in"=w415, "auto start"=TRUE, "data"=w374, "error in"=w414) -> ("task out"=w417:refnum<k21>, "error out"=w418:errorcluster)  [unwired: 9 in, 1 out]
    n196 = call-poly <vilib>:"DAQmx Write.vi"("task/channels in"=w398, "auto start"=TRUE, "data"=w372, "error in"=w397) -> ("task out"=w400:refnum<k21>, "error out"=w401:errorcluster)  [unwired: 9 in, 1 out]
    n197 = call <vilib>:"DAQmx Clear Task.vi"("task in"=w417, "error in"=w418) -> ("error out"=w412:errorcluster)  [unwired: 13 in]
    n198 = call <vilib>:"DAQmx Clear Task.vi"("task in"=w400, "error in"=w401) -> ("error out"=w395:errorcluster)  [unwired: 13 in]
    n199 = call <vilib>:"Simple Error Handler.vi"("error in (no error)"=w412) -> ()  [unwired: 4 in, 5 out]
    n200 = call <vilib>:"Simple Error Handler.vi"("error in (no error)"=w395) -> ()  [unwired: 4 in, 5 out]
    n201 = call-poly <vilib>:"DAQmx Create Virtual Channel.vi"("lines"=tag "cDAQ1Mod8/port0/line7", "line grouping"=w384) -> ("task out"=w386:refnum<k21>, "error out"=w385:errorcluster)  [unwired: 12 in]
    n202 = call-poly <vilib>:"DAQmx Create Virtual Channel.vi"("lines"=tag "cDAQ1Mod7/port0/line6", "line grouping"=w376) -> ("task out"=w378:refnum<k21>, "error out"=w377:errorcluster)  [unwired: 12 in]
    n203 = call-poly <vilib>:"DAQmx Write.vi"("task/channels in"=w386, "auto start"=TRUE, "data"=w374, "error in"=w385) -> ("task out"=w388:refnum<k21>, "error out"=w389:errorcluster)  [unwired: 9 in, 1 out]
    n204 = call-poly <vilib>:"DAQmx Write.vi"("task/channels in"=w378, "auto start"=TRUE, "data"=w372, "error in"=w377) -> ("task out"=w380:refnum<k21>, "error out"=w381:errorcluster)  [unwired: 9 in, 1 out]
    n205 = call <vilib>:"DAQmx Clear Task.vi"("task in"=w388, "error in"=w389) -> ("error out"=w383:errorcluster)  [unwired: 13 in]
    n206 = call <vilib>:"DAQmx Clear Task.vi"("task in"=w380, "error in"=w381) -> ("error out"=w375:errorcluster)  [unwired: 13 in]
    n207 = call <vilib>:"Simple Error Handler.vi"("error in (no error)"=w383) -> ()  [unwired: 4 in, 5 out]
    n208 = call <vilib>:"Simple Error Handler.vi"("error in (no error)"=w375) -> ()  [unwired: 4 in, 5 out]
  }
  n209 = control-ref of="stop"() -> (w67:refnum<vi>)
  n210 = control-ref of="XYZAER"() -> (w58:refnum<vi>)
  n211 = Obtain Queue(element data type=0.0) -> (queue out=w5:refnum<queue>)  [unwired: 4 in, 2 out]
  n212 = while {
    shift-left: 0.0 ("Plant Output") -> [w548]
    shift-right: [w543] -> _
    tunnel: w34 -> [_]
    shift-right: [w529] -> _
    shift-left: 0.01 -> [w527]
    shift-right: [w501] -> _
    shift-left: TRUE -> [w526]
    shift-right: [w503] -> _
    shift-left: w31 -> [w525]
    shift-right: [w528] -> _
    shift-left: w31 -> [w524]
    tunnel: [w498] -> w30
    tunnel: [w484] -> w15
    tunnel: w5 -> [w482]
    stop <- "Stop 8" stop-if-true
    w489 = 1 items=["one channel for each line", "one channel for all lines"] ("line grouping")
    w498 = 0.05 ("Sampling Time dt (s)")
    w507 = 1 items=["one channel for each line", "one channel for all lines"] ("line grouping")
    w515 = 0.5 ("x")
    w542 = T7 {"static gain"=2.5, "lag (s)"=2.5, "deadtime (s)"=0.01, "load"=0.0, "deadband"=0.0, "sensor noise"=0.0, "initial PV"=30.0, "plant noise"=0.0}  # Process parameters
    w544 = FALSE  # Integrator ?
    # "C."
    # "Inlet 11"
    # "Exhaust 2"
    # "B."
    # "A."
    # "A.Output to PWM Logic \nB. Simulated Plant\nC. Draw Chart"
    # "Main PID Loop Control"
    n213 = Dequeue Element(queue=w482) -> (element=w483:dbl)  [unwired: 2 in, 3 out]
    n214 = Multiply(x=w498, y=1000.0) -> (x*y=w541:dbl)
    n215 = Not(x="Autotune 8") -> (.not. x?=w545:bool)
    n216 = feedback #6() -> (w550:bool)  [unwired: 1 in]
    n217 = feedback-in #6("Autotune 8") -> ()
    n218 = Wait Until Next ms Multiple(millisecond multiple=w541) -> ()  [unwired: 1 out]
    n219 = Exclusive Or(1:w550, 2:"Autotune 8") -> (0:w549:bool)
    n220 = feedback #7() -> (w547:dbl)  [unwired: 1 in]
    n221 = Multiply(x=w483, y=-1000.0) -> (x*y=w531:dbl)
    n222 = call <vilib>:"Median PtByPt.vi"("sample length"="Median sample length 17", "x"=w531) -> ("median"=w530:dbl)  [unwired: 2 in, 1 out]
    n223 = Square(x=w530) -> (x^2=w538:dbl)
    n224 = Multiply(x=w530, y=-7.5945) -> (x*y=w534:dbl)
    n225 = Multiply(x=w538, y=0.0612) -> (x*y=w535:dbl)
    n226 = Add(x=w534, y=w535) -> (x+y=w533:dbl)
    n227 = Add(x=143.72, y=w533) -> (x+y=w496:dbl)
    n228 = case shown="False" "Autotune 8" {
      tunnel: w498 -> [w565 _]
      tunnel: [w554 w570] -> w503
      tunnel: w548 -> [_ w569]
      tunnel: "PID Gains 8" -> [w564 _]
      tunnel: "Reinitialize 8" -> [w561 _]
      tunnel: w549 -> [w563 w568]
      tunnel: w547 -> [_ w572]
      tunnel: w496 -> [w557 _]
      tunnel: "Set Point 2" -> [w556 _]
      frame False {
        # "This code is to have 'bumpless' transfer from autotuning"
        n229 = Not(x=w563) -> (.not. x?=w560:bool)
        n230 = And(x="Automatic 8", y=w560) -> (x .and. y?=w562:bool)
        n231 = call-poly <vilib>:"PID Advanced.vi"("setpoint"=w556, "auto? (T)"=w562, "manual control"="MV: 8", "process variable"=w557, "alpha"=10.0, "PID gains"=w564, "dt (s)"=w565, "reinitialize? (F)"=w561) -> ("output"=w554:dbl)  [unwired: 6 in, 1 out]
      }
      frame True {
        w575 = 10000 ("sample length")
        # "Buffering data for parameters estimation"
        n232 = call <vilib>:"Data Queue PtByPt.vi"("initial queue element"=w569, "initialize"=w568, "sample length"=w575, "input data point"=w569) -> ("Current Queue"=→"Control Output 8":dbl[])  [unwired: 3 in, 4 out]
        n233 = Select(t=0.0, s=w568, f="Excitation 8") -> (s? t:f=w573:dbl)
        n234 = Add(x=w572, y=w573) -> (x+y=w570:dbl)
        n235 = call <vilib>:"Data Queue PtByPt.vi"("initial queue element"=w570, "initialize"=w568, "sample length"=w575, "input data point"=w570) -> ("Current Queue"=→"Measurement 8":dbl[])  [unwired: 3 in, 4 out]
      }
    }
    n236 = feedback-in #7(w503, w545) -> ()
    n237 = Greater?(x=w496, y="M-2") -> (0:w484:bool)
    n238 = Add(x=w527, y=w515) -> (x+y=w516:dbl)
    n239 = Subtract(x=w527, y=w515) -> (x-y=w514:dbl)
    n240 = Equal?(x=w525, y=w503) -> (x = y?=w522:bool)
    n241 = Greater?(x=w503, y=w525) -> (0:w521:bool)
    n242 = Select(t=w526, s=w522, f=w521) -> (s? t:f=w501:bool)
    "PWM Output 8" <- w501
    n243 = call "Plant System.vi"("Integrator ?"=w544, "Plant Input"=w503, "dt (s)"=w498, "process parameters"=w542) -> ("Plant Output"=w543:dbl)  [unwired: 11 in]
    n244 = Increment(x="Set Point 2") -> (x+1=w520:dbl)
    n245 = Decrement(x="Set Point 2") -> (x-1=w519:dbl)
    n246 = Select(t=w516, s=w501, f=w514) -> (s? t:f=w529:dbl)
    n247 = Select(t=w520, s=w501, f=w519) -> (s? t:f=w518:dbl)
    n248 = Not(x=w501) -> (.not. x?=w500:bool)
    n249 = call-poly <vilib>:"DAQmx Create Virtual Channel.vi"("lines"=tag "cDAQ1Mod1/port0/line6", "line grouping"=w507) -> ("task out"=w509:refnum<k21>, "error out"=w508:errorcluster)  [unwired: 12 in]
    n250 = call-poly <vilib>:"DAQmx Create Virtual Channel.vi"("lines"=tag "cDAQ1Mod2/port0/line6", "line grouping"=w489) -> ("task out"=w491:refnum<k21>, "error out"=w490:errorcluster)  [unwired: 12 in]
    n251 = Build Array(w496, "Set Point 2", w518) -> (w517:dbl[])
    n252 = Initialize Array("INLET 2 ON/OFF 2", 1 ("dimension size")) -> (w486:bool[])
    n253 = Initialize Array(w500, 1 ("dimension size")) -> (w504:bool[])
    n254 = local write "MV: 8"(w503) -> ()
    n255 = Add(x=w524, y=w527) -> (x+y=w528:dbl)
    n256 = Build Array(w517) -> (→"Real time Data 2":dbl[][])
    n257 = call-poly <vilib>:"DAQmx Write.vi"("task/channels in"=w509, "auto start"=TRUE, "data"=w504, "error in"=w508) -> ("task out"=w511:refnum<k21>, "error out"=w512:errorcluster)  [unwired: 9 in, 1 out]
    n258 = call-poly <vilib>:"DAQmx Write.vi"("task/channels in"=w491, "auto start"=TRUE, "data"=w486, "error in"=w490) -> ("task out"=w493:refnum<k21>, "error out"=w494:errorcluster)  [unwired: 9 in, 1 out]
    n259 = call <vilib>:"DAQmx Clear Task.vi"("task in"=w511, "error in"=w512) -> ("error out"=w506:errorcluster)  [unwired: 13 in]
    n260 = call <vilib>:"DAQmx Clear Task.vi"("task in"=w493, "error in"=w494) -> ("error out"=w488:errorcluster)  [unwired: 13 in]
    n261 = call <vilib>:"Simple Error Handler.vi"("error in (no error)"=w506) -> ()  [unwired: 4 in, 5 out]
    n262 = call <vilib>:"Simple Error Handler.vi"("error in (no error)"=w488) -> ()  [unwired: 4 in, 5 out]
  }
  n263 = Obtain Queue(element data type=0.0) -> (queue out=w4:refnum<queue>)  [unwired: 4 in, 2 out]
  n264 = while {
    shift-left: 0.0 ("Plant Output") -> [w642]
    shift-right: [w637] -> _
    tunnel: w40 -> [_]
    shift-right: [w623] -> _
    shift-left: 0.01 -> [w621]
    shift-right: [w595] -> _
    shift-left: TRUE -> [w620]
    shift-right: [w597] -> _
    shift-left: w37 -> [w619]
    shift-right: [w622] -> _
    shift-left: w37 -> [w618]
    tunnel: [w592] -> w36
    tunnel: [w578] -> w14
    tunnel: w4 -> [w576]
    stop <- "Stop 7" stop-if-true
    w583 = 1 items=["one channel for each line", "one channel for all lines"] ("line grouping")
    w592 = 0.05 ("Sampling Time dt (s)")
    w601 = 1 items=["one channel for each line", "one channel for all lines"] ("line grouping")
    w609 = 0.5 ("x")
    w636 = T7 {"static gain"=2.5, "lag (s)"=2.5, "deadtime (s)"=0.01, "load"=0.0, "deadband"=0.0, "sensor noise"=0.0, "initial PV"=30.0, "plant noise"=0.0}  # Process parameters
    w638 = FALSE  # Integrator ?
    # "C."
    # "Inlet 11"
    # "Exhaust 7"
    # "B."
    # "A."
    # "A.Output to PWM Logic \nB. Simulated Plant\nC. Draw Chart"
    # "Main PID Loop Control"
    n265 = Dequeue Element(queue=w576) -> (element=w577:dbl)  [unwired: 2 in, 3 out]
    n266 = Multiply(x=w592, y=1000.0) -> (x*y=w635:dbl)
    n267 = Not(x="Autotune 7") -> (.not. x?=w639:bool)
    n268 = feedback #8() -> (w644:bool)  [unwired: 1 in]
    n269 = feedback-in #8("Autotune 7") -> ()
    n270 = Wait Until Next ms Multiple(millisecond multiple=w635) -> ()  [unwired: 1 out]
    n271 = Exclusive Or(1:w644, 2:"Autotune 7") -> (0:w643:bool)
    n272 = feedback #9() -> (w641:dbl)  [unwired: 1 in]
    n273 = Multiply(x=w577, y=-1000.0) -> (x*y=w625:dbl)
    n274 = call <vilib>:"Median PtByPt.vi"("sample length"="Median sample length 16", "x"=w625) -> ("median"=w624:dbl)  [unwired: 2 in, 1 out]
    n275 = Square(x=w624) -> (x^2=w632:dbl)
    n276 = Multiply(x=w624, y=-0.6707) -> (x*y=w628:dbl)
    n277 = Multiply(x=w632, y=0.0015) -> (x*y=w629:dbl)
    n278 = Add(x=w628, y=w629) -> (x+y=w627:dbl)
    n279 = Add(x=-0.8771, y=w627) -> (x+y=w590:dbl)
    n280 = case shown="False" "Autotune 7" {
      tunnel: w592 -> [w659 _]
      tunnel: [w648 w664] -> w597
      tunnel: w642 -> [_ w663]
      tunnel: "PID Gains 7" -> [w658 _]
      tunnel: "Reinitialize 7" -> [w655 _]
      tunnel: w643 -> [w657 w662]
      tunnel: w641 -> [_ w666]
      tunnel: w590 -> [w651 _]
      tunnel: "Set Point 7" -> [w650 _]
      frame False {
        # "This code is to have 'bumpless' transfer from autotuning"
        n281 = Not(x=w657) -> (.not. x?=w654:bool)
        n282 = And(x="Automatic 7", y=w654) -> (x .and. y?=w656:bool)
        n283 = call-poly <vilib>:"PID Advanced.vi"("setpoint"=w650, "auto? (T)"=w656, "manual control"="MV: 7", "process variable"=w651, "alpha"=10.0, "PID gains"=w658, "dt (s)"=w659, "reinitialize? (F)"=w655) -> ("output"=w648:dbl)  [unwired: 6 in, 1 out]
      }
      frame True {
        w669 = 10000 ("sample length")
        # "Buffering data for parameters estimation"
        n284 = call <vilib>:"Data Queue PtByPt.vi"("initial queue element"=w663, "initialize"=w662, "sample length"=w669, "input data point"=w663) -> ("Current Queue"=→"Control Output 7":dbl[])  [unwired: 3 in, 4 out]
        n285 = Select(t=0.0, s=w662, f="Excitation 7") -> (s? t:f=w667:dbl)
        n286 = Add(x=w666, y=w667) -> (x+y=w664:dbl)
        n287 = call <vilib>:"Data Queue PtByPt.vi"("initial queue element"=w664, "initialize"=w662, "sample length"=w669, "input data point"=w664) -> ("Current Queue"=→"Measurement 7":dbl[])  [unwired: 3 in, 4 out]
      }
    }
    n288 = feedback-in #9(w597, w639) -> ()
    n289 = Greater?(x=w590, y="M-7") -> (0:w578:bool)
    n290 = Add(x=w621, y=w609) -> (x+y=w610:dbl)
    n291 = Subtract(x=w621, y=w609) -> (x-y=w608:dbl)
    n292 = Equal?(x=w619, y=w597) -> (x = y?=w616:bool)
    n293 = Greater?(x=w597, y=w619) -> (0:w615:bool)
    n294 = Select(t=w620, s=w616, f=w615) -> (s? t:f=w595:bool)
    "PWM Output 7" <- w595
    n295 = call "Plant System.vi"("Integrator ?"=w638, "Plant Input"=w597, "dt (s)"=w592, "process parameters"=w636) -> ("Plant Output"=w637:dbl)  [unwired: 11 in]
    n296 = Increment(x="Set Point 7") -> (x+1=w614:dbl)
    n297 = Decrement(x="Set Point 7") -> (x-1=w613:dbl)
    n298 = Select(t=w610, s=w595, f=w608) -> (s? t:f=w623:dbl)
    n299 = Select(t=w614, s=w595, f=w613) -> (s? t:f=w612:dbl)
    n300 = Not(x=w595) -> (.not. x?=w594:bool)
    n301 = call-poly <vilib>:"DAQmx Create Virtual Channel.vi"("lines"=tag "cDAQ1Mod8/port0/line4", "line grouping"=w601) -> ("task out"=w603:refnum<k21>, "error out"=w602:errorcluster)  [unwired: 12 in]
    n302 = call-poly <vilib>:"DAQmx Create Virtual Channel.vi"("lines"=tag "cDAQ1Mod7/port0/line3", "line grouping"=w583) -> ("task out"=w585:refnum<k21>, "error out"=w584:errorcluster)  [unwired: 12 in]
    n303 = Build Array(w590, "Set Point 7", w612) -> (w611:dbl[])
    n304 = Initialize Array("INLET 7 ON/OFF 2", 1 ("dimension size")) -> (w580:bool[])
    n305 = Initialize Array(w594, 1 ("dimension size")) -> (w598:bool[])
    n306 = local write "MV: 7"(w597) -> ()
    n307 = Add(x=w618, y=w621) -> (x+y=w622:dbl)
    n308 = Build Array(w611) -> (→"Real time Data 7":dbl[][])
    n309 = call-poly <vilib>:"DAQmx Write.vi"("task/channels in"=w603, "auto start"=TRUE, "data"=w598, "error in"=w602) -> ("task out"=w605:refnum<k21>, "error out"=w606:errorcluster)  [unwired: 9 in, 1 out]
    n310 = call-poly <vilib>:"DAQmx Write.vi"("task/channels in"=w585, "auto start"=TRUE, "data"=w580, "error in"=w584) -> ("task out"=w587:refnum<k21>, "error out"=w588:errorcluster)  [unwired: 9 in, 1 out]
    n311 = call <vilib>:"DAQmx Clear Task.vi"("task in"=w605, "error in"=w606) -> ("error out"=w600:errorcluster)  [unwired: 13 in]
    n312 = call <vilib>:"DAQmx Clear Task.vi"("task in"=w587, "error in"=w588) -> ("error out"=w582:errorcluster)  [unwired: 13 in]
    n313 = call <vilib>:"Simple Error Handler.vi"("error in (no error)"=w600) -> ()  [unwired: 4 in, 5 out]
    n314 = call <vilib>:"Simple Error Handler.vi"("error in (no error)"=w582) -> ()  [unwired: 4 in, 5 out]
  }
  n315 = Obtain Queue(element data type=0.0) -> (queue out=w10:refnum<queue>)  [unwired: 4 in, 2 out]
  n316 = while {
    shift-left: 0.0 ("Plant Output") -> [w769]
    shift-right: [w764] -> _
    tunnel: w88 -> [_]
    shift-right: [w750] -> _
    shift-left: 0.01 -> [w748]
    shift-right: [w723] -> _
    shift-left: TRUE -> [w747]
    shift-right: [w725] -> _
    shift-left: w85 -> [w746]
    shift-right: [w749] -> _
    shift-left: w85 -> [w745]
    tunnel: [w720] -> w84
    tunnel: [w717] -> w1
    tunnel: w12 -> [w694]
    tunnel: w10 -> [w693]
    tunnel: w8 -> [w692]
    tunnel: w5 -> [w689]
    tunnel: w4 -> [w688]
    stop <- "Stop" stop-if-true
    w673 = 1 items=["one channel for each line", "one channel for all lines"] ("line grouping")
    w681 = 1 items=["one channel for each line", "one channel for all lines"] ("line grouping")
    w710 = 1 items=["one channel for each line", "one channel for all lines"] ("line grouping")
    w720 = 0.05 ("Sampling Time dt (s)")
    w728 = 1 items=["one channel for each line", "one channel for all lines"] ("line grouping")
    w736 = 0.5 ("x")
    w763 = T7 {"static gain"=2.5, "lag (s)"=2.5, "deadtime (s)"=0.01, "load"=0.0, "deadband"=0.0, "sensor noise"=0.0, "initial PV"=30.0, "plant noise"=0.0}  # Process parameters
    w765 = FALSE  # Integrator ?
    # "Inlet 11"
    # "Exhaust 12"
    # "C."
    # "Inlet 11"
    # "Exhaust 11"
    # "B."
    # "A."
    # "A.Output to PWM Logic \nB. Simulated Plant\nC. Draw Chart"
    # "Main PID Loop Control"
    n317 = call-poly <vilib>:"DAQmx Read.vi"("task/channels in"=refnum<k21> "1_4_2_7_6_5") -> ("data"=w700:dbl[])  [unwired: 12 in, 2 out]
    n318 = Index Array(array=w700, index=0) -> (element=w695:dbl)
    n319 = Index Array(array=w700, index=1) -> (element=w696:dbl)
    n320 = Index Array(array=w700, index=2) -> (element=w691:dbl)
    n321 = Index Array(array=w700, index=5) -> (element=w698:dbl)
    n322 = Index Array(array=w700, index=4) -> (element=w697:dbl)
    n323 = Index Array(array=w700, index=3) -> (element=w690:dbl)
    n324 = Enqueue Element(queue=w693, element=w695) -> ()  [unwired: 2 in, 3 out]
    n325 = Enqueue Element(queue=w689, element=w691) -> ()  [unwired: 2 in, 3 out]
    n326 = Multiply(x=w720, y=1000.0) -> (x*y=w762:dbl)
    n327 = Enqueue Element(queue=w692, element=w696) -> ()  [unwired: 2 in, 3 out]
    n328 = Not(x="Autotune") -> (.not. x?=w766:bool)
    n329 = feedback #10() -> (w771:bool)  [unwired: 1 in]
    n330 = feedback-in #10("Autotune") -> ()
    n331 = Enqueue Element(queue=w688, element=w690) -> ()  [unwired: 2 in, 3 out]
    n332 = Wait Until Next ms Multiple(millisecond multiple=w762) -> ()  [unwired: 1 out]
    n333 = Exclusive Or(1:w771, 2:"Autotune") -> (0:w770:bool)
    n334 = feedback #11() -> (w768:dbl)  [unwired: 1 in]
    n335 = Enqueue Element(queue=w694, element=w697) -> ()  [unwired: 2 in, 3 out]
    n336 = Multiply(x=w698, y=-1000.0) -> (x*y=w752:dbl)
    n337 = call <vilib>:"Median PtByPt.vi"("sample length"="Median sample length", "x"=w752) -> ("median"=w751:dbl)  [unwired: 2 in, 1 out]
    n338 = Square(x=w751) -> (x^2=w759:dbl)
    n339 = Multiply(x=w751, y=-39.646) -> (x*y=w755:dbl)
    n340 = Multiply(x=w759, y=0.2324) -> (x*y=w756:dbl)
    n341 = Add(x=w755, y=w756) -> (x+y=w754:dbl)
    n342 = Add(x=1678.0, y=w754) -> (x+y=w718:dbl)
    n343 = case shown="False" "Autotune" {
      tunnel: w720 -> [w786 _]
      tunnel: [w775 w791] -> w725
      tunnel: w769 -> [_ w790]
      tunnel: "PID Gains" -> [w785 _]
      tunnel: "Reinitialize" -> [w782 _]
      tunnel: w770 -> [w784 w789]
      tunnel: w768 -> [_ w793]
      tunnel: w718 -> [w778 _]
      tunnel: "Set Point 11,12" -> [w777 _]
      frame False {
        # "This code is to have 'bumpless' transfer from autotuning"
        n344 = Not(x=w784) -> (.not. x?=w781:bool)
        n345 = And(x="Automatic", y=w781) -> (x .and. y?=w783:bool)
        n346 = call-poly <vilib>:"PID Advanced.vi"("setpoint"=w777, "auto? (T)"=w783, "manual control"="MV:", "process variable"=w778, "alpha"=10.0, "PID gains"=w785, "dt (s)"=w786, "reinitialize? (F)"=w782) -> ("output"=w775:dbl)  [unwired: 6 in, 1 out]
      }
      frame True {
        w796 = 10000 ("sample length")
        # "Buffering data for parameters estimation"
        n347 = call <vilib>:"Data Queue PtByPt.vi"("initial queue element"=w790, "initialize"=w789, "sample length"=w796, "input data point"=w790) -> ("Current Queue"=→"Control Output":dbl[])  [unwired: 3 in, 4 out]
        n348 = Select(t=0.0, s=w789, f="Excitation") -> (s? t:f=w794:dbl)
        n349 = Add(x=w793, y=w794) -> (x+y=w791:dbl)
        n350 = call <vilib>:"Data Queue PtByPt.vi"("initial queue element"=w791, "initialize"=w789, "sample length"=w796, "input data point"=w791) -> ("Current Queue"=→"Measurement":dbl[])  [unwired: 3 in, 4 out]
      }
    }
    n351 = feedback-in #11(w725, w766) -> ()
    n352 = Greater?(x=w718, y="M-11,12") -> (0:w717:bool)
    n353 = Add(x=w748, y=w736) -> (x+y=w737:dbl)
    n354 = Subtract(x=w748, y=w736) -> (x-y=w735:dbl)
    n355 = Equal?(x=w746, y=w725) -> (x = y?=w743:bool)
    n356 = Greater?(x=w725, y=w746) -> (0:w742:bool)
    n357 = Select(t=w747, s=w743, f=w742) -> (s? t:f=w723:bool)
    "PWM Output" <- w723
    n358 = call "Plant System.vi"("Integrator ?"=w765, "Plant Input"=w725, "dt (s)"=w720, "process parameters"=w763) -> ("Plant Output"=w764:dbl)  [unwired: 11 in]
    n359 = Increment(x="Set Point 11,12") -> (x+1=w741:dbl)
    n360 = Decrement(x="Set Point 11,12") -> (x-1=w740:dbl)
    n361 = Select(t=w737, s=w723, f=w735) -> (s? t:f=w750:dbl)
    n362 = Select(t=w741, s=w723, f=w740) -> (s? t:f=w739:dbl)
    n363 = Not(x=w723) -> (.not. x?=w722:bool)
    n364 = call-poly <vilib>:"DAQmx Create Virtual Channel.vi"("lines"=tag "cDAQ1Mod1/port0/line2", "line grouping"=w728) -> ("task out"=w730:refnum<k21>, "error out"=w729:errorcluster)  [unwired: 12 in]
    n365 = call-poly <vilib>:"DAQmx Create Virtual Channel.vi"("lines"=tag "cDAQ1Mod2/port0/line2", "line grouping"=w710) -> ("task out"=w712:refnum<k21>, "error out"=w711:errorcluster)  [unwired: 12 in]
    n366 = Build Array(w718, "Set Point 11,12", w739) -> (w738:dbl[])
    n367 = Initialize Array("INLET", 1 ("dimension size")) -> (w670:bool[])
    n368 = Initialize Array(w722, 1 ("dimension size")) -> (w671:bool[])
    n369 = call-poly <vilib>:"DAQmx Create Virtual Channel.vi"("lines"=tag "cDAQ1Mod8/port0/line2", "line grouping"=w681) -> ("task out"=w683:refnum<k21>, "error out"=w682:errorcluster)  [unwired: 12 in]
    n370 = call-poly <vilib>:"DAQmx Create Virtual Channel.vi"("lines"=tag "cDAQ1Mod7/port0/line1", "line grouping"=w673) -> ("task out"=w675:refnum<k21>, "error out"=w674:errorcluster)  [unwired: 12 in]
    n371 = local write "MV:"(w725) -> ()
    n372 = Add(x=w745, y=w748) -> (x+y=w749:dbl)
    n373 = Build Array(w738) -> (→"Real time Data -11,12":dbl[][])
    n374 = call-poly <vilib>:"DAQmx Write.vi"("task/channels in"=w730, "auto start"=TRUE, "data"=w671, "error in"=w729) -> ("task out"=w732:refnum<k21>, "error out"=w733:errorcluster)  [unwired: 9 in, 1 out]
    n375 = call-poly <vilib>:"DAQmx Write.vi"("task/channels in"=w712, "auto start"=TRUE, "data"=w670, "error in"=w711) -> ("task out"=w714:refnum<k21>, "error out"=w715:errorcluster)  [unwired: 9 in, 1 out]
    n376 = call-poly <vilib>:"DAQmx Write.vi"("task/channels in"=w683, "auto start"=TRUE, "data"=w671, "error in"=w682) -> ("task out"=w685:refnum<k21>, "error out"=w686:errorcluster)  [unwired: 9 in, 1 out]
    n377 = call-poly <vilib>:"DAQmx Write.vi"("task/channels in"=w675, "auto start"=TRUE, "data"=w670, "error in"=w674) -> ("task out"=w677:refnum<k21>, "error out"=w678:errorcluster)  [unwired: 9 in, 1 out]
    n378 = call <vilib>:"DAQmx Clear Task.vi"("task in"=w732, "error in"=w733) -> ("error out"=w727:errorcluster)  [unwired: 13 in]
    n379 = call <vilib>:"DAQmx Clear Task.vi"("task in"=w714, "error in"=w715) -> ("error out"=w709:errorcluster)  [unwired: 13 in]
    n380 = call <vilib>:"DAQmx Clear Task.vi"("task in"=w685, "error in"=w686) -> ("error out"=w680:errorcluster)  [unwired: 13 in]
    n381 = call <vilib>:"DAQmx Clear Task.vi"("task in"=w677, "error in"=w678) -> ("error out"=w672:errorcluster)  [unwired: 13 in]
    n382 = call <vilib>:"Simple Error Handler.vi"("error in (no error)"=w727) -> ()  [unwired: 4 in, 5 out]
    n383 = call <vilib>:"Simple Error Handler.vi"("error in (no error)"=w709) -> ()  [unwired: 4 in, 5 out]
    n384 = call <vilib>:"Simple Error Handler.vi"("error in (no error)"=w680) -> ()  [unwired: 4 in, 5 out]
    n385 = call <vilib>:"Simple Error Handler.vi"("error in (no error)"=w672) -> ()  [unwired: 4 in, 5 out]
  }
  n386 = while {
    tunnel: w88 -> [_]
    tunnel: w84 -> [w800]
    stop <- w810 stop-if-true
    # "If dT and deadtime have similar values, the identification could evaluate deadtime as zero and this generates proportional gain equal to Inf. This code avoid gain changes in this situations."
    # "Autotuning Loop"
    n387 = local read "Control Output"() -> (w812:dbl[])
    n388 = local read "Measurement"() -> (w811:dbl[])
    n389 = case shown="\"Chien-Hrones-Reswick\"" "Control" {
      tunnel: w812 -> [w821 w829 w838 w847]
      tunnel: w811 -> [w820 w828 w837 w846]
      tunnel: [w819 w827 w836 w845] -> w799
      tunnel: [w818 w826 w835 w844] -> w798
      tunnel: w800 -> [w817 w825 w834 w843]
      tunnel: [w816 w824 w833 w842] -> w797
      tunnel: [w815 w823 w832 w841] -> w802
      tunnel: "Type of controller" -> [w814 w822 w831 w840]
      frame "Ziegler-Nichols", Default {
        n390 = call-poly <vilib>:"PID Autotuning Design.vi"("Ziegler-Nichols Speed"="Ziegler-Nichols speed", "Type of Controller"=w814, "dt (s)"=w817, "Response signal"=w820, "Stimulus signal"=w821) -> ("PID gains"=w815:T3, "response operating point"=w818:dbl, "stimulus operating point"=w819:dbl, "Plant Parameters"=w816:T5)  [unwired: 3 in]
      }
      frame "Cohen-Coon" {
        n391 = call-poly <vilib>:"PID Autotuning Design.vi"("Type of Controller"=w822, "dt (s)"=w825, "Response signal"=w828, "Stimulus signal"=w829) -> ("PID gains"=w823:T3, "response offset"=w826:dbl, "stimulus offset"=w827:dbl, "Plant Parameters"=w824:T5)  [unwired: 4 in]
      }
      frame "Chien-Hrones-Reswick" {
        n392 = call-poly <vilib>:"PID Autotuning Design.vi"("Tuning specifications"="Tuning specifications", "Type of Controller"=w831, "dt (s)"=w834, "Response signal"=w837, "Stimulus signal"=w838) -> ("PID gains"=w832:T3, "response offset"=w835:dbl, "stimulus offset"=w836:dbl, "Plant Parameters"=w833:T5)  [unwired: 3 in]
      }
      frame "Internal Model Control" {
        n393 = call-poly <vilib>:"PID Autotuning Design.vi"("Desired Time Constant (tau_c)"="Multiplicative factor", "Type of Controller"=w840, "dt (s)"=w843, "Response signal"=w846, "Stimulus signal"=w847) -> ("PID gains"=w841:T3, "response offset"=w844:dbl, "stimulus offset"=w845:dbl, "Plant Parameters"=w842:T5)  [unwired: 3 in]
      }
    }
    "Stimulus operating point" <- w799
    "Response operating point" <- w798
    "Identified Plant Parameters" <- w797
    n394 = Unbundle(w802) -> ("proportional gain (Kc)"=w805:dbl)  [unwired: 2 out]
    n395 = Equal?(x=w805, y=inf) -> (x = y?=w804:bool)
    n396 = feedback #12() -> (w803:T3)  [unwired: 1 in]
    n397 = Select(t=w803, s=w804, f=w802) -> (s? t:f=w801:T3)
    "Tuned PID gains" <- w801
    n398 = feedback-in #12(w801) -> ()
    n399 = case shown="True" "Accept gain" {
      tunnel: w801 -> [_ w848]
      frame False {
      }
      frame True {
        n400 = local write "PID Gains"(w848) -> ()
      }
    }
    n401 = local read "Stop"() -> (w810:bool)
  }
  n402 = while {
    shift-left: 0.0 ("Plant Output") -> [w933]
    shift-right: [w928] -> _
    tunnel: w22 -> [_]
    shift-right: [w914] -> _
    shift-left: 0.01 -> [w912]
    shift-right: [w887] -> _
    shift-left: TRUE -> [w911]
    shift-right: [w889] -> _
    shift-left: w19 -> [w910]
    shift-right: [w913] -> _
    shift-left: w19 -> [w909]
    tunnel: [w884] -> w18
    tunnel: [w871] -> w3
    tunnel: w10 -> [w869]
    stop <- "Stop 12" stop-if-true
    w854 = 1 items=["one channel for each line", "one channel for all lines"] ("line grouping")
    w862 = 1 items=["one channel for each line", "one channel for all lines"] ("line grouping")
    w875 = 1 items=["one channel for each line", "one channel for all lines"] ("line grouping")
    w884 = 0.05 ("Sampling Time dt (s)")
    w892 = 1 items=["one channel for each line", "one channel for all lines"] ("line grouping")
    w900 = 0.5 ("x")
    w927 = T7 {"static gain"=2.5, "lag (s)"=2.5, "deadtime (s)"=0.01, "load"=0.0, "deadband"=0.0, "sensor noise"=0.0, "initial PV"=30.0, "plant noise"=0.0}  # Process parameters
    w929 = FALSE  # Integrator ?
    # "Inlet 11"
    # "Exhaust 5"
    # "C."
    # "Inlet 11"
    # "Exhaust 1"
    # "B."
    # "A."
    # "A.Output to PWM Logic \nB. Simulated Plant\nC. Draw Chart"
    # "Main PID Loop Control"
    n403 = Dequeue Element(queue=w869) -> (element=w870:dbl)  [unwired: 2 in, 3 out]
    n404 = Multiply(x=w884, y=1000.0) -> (x*y=w926:dbl)
    n405 = Not(x="Autotune 12") -> (.not. x?=w930:bool)
    n406 = feedback #13() -> (w935:bool)  [unwired: 1 in]
    n407 = feedback-in #13("Autotune 12") -> ()
    n408 = Wait Until Next ms Multiple(millisecond multiple=w926) -> ()  [unwired: 1 out]
    n409 = Exclusive Or(1:w935, 2:"Autotune 12") -> (0:w934:bool)
    n410 = feedback #14() -> (w932:dbl)  [unwired: 1 in]
    n411 = Multiply(x=w870, y=-1000.0) -> (x*y=w916:dbl)
    n412 = call <vilib>:"Median PtByPt.vi"("sample length"="Median sample length 21", "x"=w916) -> ("median"=w915:dbl)  [unwired: 2 in, 1 out]
    n413 = Square(x=w915) -> (x^2=w923:dbl)
    n414 = Multiply(x=w915, y=2.7367) -> (x*y=w919:dbl)
    n415 = Multiply(x=w923, y=0.0108) -> (x*y=w920:dbl)
    n416 = Add(x=w919, y=w920) -> (x+y=w918:dbl)
    n417 = Add(x=-331.61, y=w918) -> (x+y=w882:dbl)
    n418 = case shown="True" "Autotune 12" {
      tunnel: w884 -> [w950 _]
      tunnel: [w939 w955] -> w889
      tunnel: w933 -> [_ w954]
      tunnel: "PID Gains 12" -> [w949 _]
      tunnel: "Reinitialize 12" -> [w946 _]
      tunnel: w934 -> [w948 w953]
      tunnel: w932 -> [_ w957]
      tunnel: w882 -> [w942 _]
      tunnel: "Set Point 1,5" -> [w941 _]
      frame False {
        # "This code is to have 'bumpless' transfer from autotuning"
        n419 = Not(x=w948) -> (.not. x?=w945:bool)
        n420 = And(x="Automatic 12", y=w945) -> (x .and. y?=w947:bool)
        n421 = call-poly <vilib>:"PID Advanced.vi"("setpoint"=w941, "auto? (T)"=w947, "manual control"="MV: 12", "process variable"=w942, "alpha"=10.0, "PID gains"=w949, "dt (s)"=w950, "reinitialize? (F)"=w946) -> ("output"=w939:dbl)  [unwired: 6 in, 1 out]
      }
      frame True {
        w960 = 10000 ("sample length")
        # "Buffering data for parameters estimation"
        n422 = call <vilib>:"Data Queue PtByPt.vi"("initial queue element"=w954, "initialize"=w953, "sample length"=w960, "input data point"=w954) -> ("Current Queue"=→"Control Output 12":dbl[])  [unwired: 3 in, 4 out]
        n423 = Select(t=0.0, s=w953, f="Excitation 12") -> (s? t:f=w958:dbl)
        n424 = Add(x=w957, y=w958) -> (x+y=w955:dbl)
        n425 = call <vilib>:"Data Queue PtByPt.vi"("initial queue element"=w955, "initialize"=w953, "sample length"=w960, "input data point"=w955) -> ("Current Queue"=→"Measurement 12":dbl[])  [unwired: 3 in, 4 out]
      }
    }
    n426 = feedback-in #14(w889, w930) -> ()
    n427 = Greater?(x=w882, y="M-1,5") -> (0:w871:bool)
    n428 = Add(x=w912, y=w900) -> (x+y=w901:dbl)
    n429 = Subtract(x=w912, y=w900) -> (x-y=w899:dbl)
    n430 = Equal?(x=w910, y=w889) -> (x = y?=w907:bool)
    n431 = Greater?(x=w889, y=w910) -> (0:w906:bool)
    n432 = Select(t=w911, s=w907, f=w906) -> (s? t:f=w887:bool)
    "PWM Output 12" <- w887
    n433 = call "Plant System.vi"("Integrator ?"=w929, "Plant Input"=w889, "dt (s)"=w884, "process parameters"=w927) -> ("Plant Output"=w928:dbl)  [unwired: 11 in]
    n434 = Increment(x="Set Point 1,5") -> (x+1=w905:dbl)
    n435 = Decrement(x="Set Point 1,5") -> (x-1=w904:dbl)
    n436 = Select(t=w901, s=w887, f=w899) -> (s? t:f=w914:dbl)
    n437 = Select(t=w905, s=w887, f=w904) -> (s? t:f=w903:dbl)
    n438 = Not(x=w887) -> (.not. x?=w886:bool)
    n439 = call-poly <vilib>:"DAQmx Create Virtual Channel.vi"("lines"=tag "cDAQ1Mod1/port0/line7", "line grouping"=w892) -> ("task out"=w894:refnum<k21>, "error out"=w893:errorcluster)  [unwired: 12 in]
    n440 = call-poly <vilib>:"DAQmx Create Virtual Channel.vi"("lines"=tag "cDAQ1Mod2/port0/line7", "line grouping"=w875) -> ("task out"=w877:refnum<k21>, "error out"=w876:errorcluster)  [unwired: 12 in]
    n441 = Build Array(w882, "Set Point 1,5", w903) -> (w902:dbl[])
    n442 = Initialize Array("INLET 1,5 ON/OFF 3", 1 ("dimension size")) -> (w872:bool[])
    n443 = Initialize Array(w886, 1 ("dimension size")) -> (w849:bool[])
    n444 = local write "MV: 12"(w889) -> ()
    n445 = Add(x=w909, y=w912) -> (x+y=w913:dbl)
    n446 = Build Array(w902) -> (→"Real time Data 1,5":dbl[][])
    n447 = call-poly <vilib>:"DAQmx Write.vi"("task/channels in"=w894, "auto start"=TRUE, "data"=w849, "error in"=w893) -> ("task out"=w896:refnum<k21>, "error out"=w897:errorcluster)  [unwired: 9 in, 1 out]
    n448 = call-poly <vilib>:"DAQmx Write.vi"("task/channels in"=w877, "auto start"=TRUE, "data"=w872, "error in"=w876) -> ("task out"=w879:refnum<k21>, "error out"=w880:errorcluster)  [unwired: 9 in, 1 out]
    n449 = call <vilib>:"DAQmx Clear Task.vi"("task in"=w896, "error in"=w897) -> ("error out"=w891:errorcluster)  [unwired: 13 in]
    n450 = call <vilib>:"DAQmx Clear Task.vi"("task in"=w879, "error in"=w880) -> ("error out"=w874:errorcluster)  [unwired: 13 in]
    n451 = call <vilib>:"Simple Error Handler.vi"("error in (no error)"=w891) -> ()  [unwired: 4 in, 5 out]
    n452 = call <vilib>:"Simple Error Handler.vi"("error in (no error)"=w874) -> ()  [unwired: 4 in, 5 out]
    n453 = call-poly <vilib>:"DAQmx Create Virtual Channel.vi"("lines"=tag "cDAQ1Mod1/port0/line5", "line grouping"=w862) -> ("task out"=w864:refnum<k21>, "error out"=w863:errorcluster)  [unwired: 12 in]
    n454 = call-poly <vilib>:"DAQmx Create Virtual Channel.vi"("lines"=tag "cDAQ1Mod2/port0/line5", "line grouping"=w854) -> ("task out"=w856:refnum<k21>, "error out"=w855:errorcluster)  [unwired: 12 in]
    n455 = Initialize Array("INLET 1,5 ON/OFF 3", 1 ("dimension size")) -> (w851:bool[])
    n456 = call-poly <vilib>:"DAQmx Write.vi"("task/channels in"=w864, "auto start"=TRUE, "data"=w849, "error in"=w863) -> ("task out"=w866:refnum<k21>, "error out"=w867:errorcluster)  [unwired: 9 in, 1 out]
    n457 = call-poly <vilib>:"DAQmx Write.vi"("task/channels in"=w856, "auto start"=TRUE, "data"=w851, "error in"=w855) -> ("task out"=w858:refnum<k21>, "error out"=w859:errorcluster)  [unwired: 9 in, 1 out]
    n458 = call <vilib>:"DAQmx Clear Task.vi"("task in"=w866, "error in"=w867) -> ("error out"=w861:errorcluster)  [unwired: 13 in]
    n459 = call <vilib>:"DAQmx Clear Task.vi"("task in"=w858, "error in"=w859) -> ("error out"=w853:errorcluster)  [unwired: 13 in]
    n460 = call <vilib>:"Simple Error Handler.vi"("error in (no error)"=w861) -> ()  [unwired: 4 in, 5 out]
    n461 = call <vilib>:"Simple Error Handler.vi"("error in (no error)"=w853) -> ()  [unwired: 4 in, 5 out]
  }
  n462 = Compound Arithmetic op=OR(w1, w2, w3, w16, w15, w14) -> (w17:bool)
  "?" <- w17
  n463 = case shown="True" w17 {
    frame False {
    }
    frame True {
      n464 = call <vilib>:"Beep.vi"("use system alert? (T)"=FALSE, "duration (msec)"=u32 2000, "frequency (Hz)"=u32 15000) -> ()  [unwired: 9 in]
    }
  }
  n465 = control-ref of="PnoData"() -> (w49:refnum<vi>)
  n466 = call <instrlib>:"PDI data xyzaer loop.vi"("Data Ready Refnum"=w49, "FrameCount Ctl Ref"=w59, "error in (no error)"=w69, "xyzaer array\nRefnum"=w58, "Stop Ctl Ref"=w67, "pDev"=w68) -> ("error out"=w56:errorcluster, "Loop Iter"=w60:i32, "dup pDev"=w57:u32)  [unwired: 3 out]
  n467 = local write "Loop Iter"(w60) -> ()
  n468 = local write "Stop 9"(w28) -> ()
  n469 = local write "Stop 12"(w22) -> ()
  n470 = call <instrlib>:"PDI action stopcont.vi"("error in (no error)"=w56, "pDev"=w57) -> ("error out"=w65:errorcluster, "Running"=w70:bool, "dup pDev"=w71:u32)  [unwired: 7 out]
  n471 = local write "Stop 8"(w34) -> ()
  n472 = local write "Stop 7"(w40) -> ()
  n473 = local write "Running"(w70) -> ()
  n474 = case shown="No Error" w56 {
    tunnel: w64 -> [w964 _]
    frame No Error {
      # "Success up to here"
      n475 = call "Elapsed Time"("Set Start Time (s)"=w964) -> ("Present Text"=w966:string, "Elapsed Time Text"=w965:string)  [unwired: 4 in, 13 out]
      n476 = local write "Stop Time Text"(w966) -> ()
      n477 = local write "Elapsed Time Text"(w965) -> ()
    }
    frame Error {
      # "Error somewhere;\nStop Time is irrelevant"
    }
  }
  n478 = while {
    tunnel: w28 -> [_]
    tunnel: w24 -> [w970]
    stop <- w980 stop-if-true
    # "If dT and deadtime have similar values, the identification could evaluate deadtime as zero and this generates proportional gain equal to Inf. This code avoid gain changes in this situations."
    # "Autotuning Loop"
    n479 = local read "Control Output 9"() -> (w982:dbl[])
    n480 = local read "Measurement 9"() -> (w981:dbl[])
    n481 = case shown="\"Internal Model Control\"" "Control 9" {
      tunnel: w982 -> [w991 w999 w1008 w1017]
      tunnel: w981 -> [w990 w998 w1007 w1016]
      tunnel: [w989 w997 w1006 w1015] -> w968
      tunnel: [w988 w996 w1005 w1014] -> w967
      tunnel: w970 -> [w987 w995 w1004 w1013]
      tunnel: [w986 w994 w1003 w1012] -> w969
      tunnel: [w985 w993 w1002 w1011] -> w972
      tunnel: "Type of controller 9" -> [w984 w992 w1001 w1010]
      frame "Ziegler-Nichols", Default {
        n482 = call-poly <vilib>:"PID Autotuning Design.vi"("Ziegler-Nichols Speed"="Ziegler-Nichols speed 9", "Type of Controller"=w984, "dt (s)"=w987, "Response signal"=w990, "Stimulus signal"=w991) -> ("PID gains"=w985:T3, "response operating point"=w988:dbl, "stimulus operating point"=w989:dbl, "Plant Parameters"=w986:T5)  [unwired: 3 in]
      }
      frame "Cohen-Coon" {
        n483 = call-poly <vilib>:"PID Autotuning Design.vi"("Type of Controller"=w992, "dt (s)"=w995, "Response signal"=w998, "Stimulus signal"=w999) -> ("PID gains"=w993:T3, "response offset"=w996:dbl, "stimulus offset"=w997:dbl, "Plant Parameters"=w994:T5)  [unwired: 4 in]
      }
      frame "Chien-Hrones-Reswick" {
        n484 = call-poly <vilib>:"PID Autotuning Design.vi"("Tuning specifications"="Tuning specifications 9", "Type of Controller"=w1001, "dt (s)"=w1004, "Response signal"=w1007, "Stimulus signal"=w1008) -> ("PID gains"=w1002:T3, "response offset"=w1005:dbl, "stimulus offset"=w1006:dbl, "Plant Parameters"=w1003:T5)  [unwired: 3 in]
      }
      frame "Internal Model Control" {
        n485 = call-poly <vilib>:"PID Autotuning Design.vi"("Desired Time Constant (tau_c)"="Multiplicative factor 9", "Type of Controller"=w1010, "dt (s)"=w1013, "Response signal"=w1016, "Stimulus signal"=w1017) -> ("PID gains"=w1011:T3, "response offset"=w1014:dbl, "stimulus offset"=w1015:dbl, "Plant Parameters"=w1012:T5)  [unwired: 3 in]
      }
    }
    "Identified Plant Parameters 9" <- w969
    "Response operating point 9" <- w967
    "Stimulus operating point 9" <- w968
    n486 = Unbundle(w972) -> ("proportional gain (Kc)"=w975:dbl)  [unwired: 2 out]
    n487 = Equal?(x=w975, y=inf) -> (x = y?=w974:bool)
    n488 = feedback #15() -> (w973:T3)  [unwired: 1 in]
    n489 = Select(t=w973, s=w974, f=w972) -> (s? t:f=w971:T3)
    "Tuned PID gains 9" <- w971
    n490 = feedback-in #15(w971) -> ()
    n491 = case shown="True" "Accept gain 9" {
      tunnel: w971 -> [_ w1018]
      frame False {
      }
      frame True {
        n492 = local write "PID Gains 9"(w1018) -> ()
      }
    }
    n493 = local read "Stop 9"() -> (w980:bool)
  }
  n494 = while {
    tunnel: w22 -> [_]
    tunnel: w18 -> [w1022]
    stop <- w1032 stop-if-true
    # "If dT and deadtime have similar values, the identification could evaluate deadtime as zero and this generates proportional gain equal to Inf. This code avoid gain changes in this situations."
    # "Autotuning Loop"
    n495 = local read "Control Output 12"() -> (w1034:dbl[])
    n496 = local read "Measurement 12"() -> (w1033:dbl[])
    n497 = case shown="\"Ziegler-Nichols\", Default" "Control 12" {
      tunnel: w1034 -> [w1043 w1051 w1060 w1069]
      tunnel: w1033 -> [w1042 w1050 w1059 w1068]
      tunnel: [w1041 w1049 w1058 w1067] -> w1020
      tunnel: [w1040 w1048 w1057 w1066] -> w1021
      tunnel: w1022 -> [w1039 w1047 w1056 w1065]
      tunnel: [w1038 w1046 w1055 w1064] -> w1019
      tunnel: [w1037 w1045 w1054 w1063] -> w1024
      tunnel: "Type of controller 12" -> [w1036 w1044 w1053 w1062]
      frame "Ziegler-Nichols", Default {
        n498 = call-poly <vilib>:"PID Autotuning Design.vi"("Ziegler-Nichols Speed"="Ziegler-Nichols speed 12", "Type of Controller"=w1036, "dt (s)"=w1039, "Response signal"=w1042, "Stimulus signal"=w1043) -> ("PID gains"=w1037:T3, "response operating point"=w1040:dbl, "stimulus operating point"=w1041:dbl, "Plant Parameters"=w1038:T5)  [unwired: 3 in]
      }
      frame "Cohen-Coon" {
        n499 = call-poly <vilib>:"PID Autotuning Design.vi"("Type of Controller"=w1044, "dt (s)"=w1047, "Response signal"=w1050, "Stimulus signal"=w1051) -> ("PID gains"=w1045:T3, "response offset"=w1048:dbl, "stimulus offset"=w1049:dbl, "Plant Parameters"=w1046:T5)  [unwired: 4 in]
      }
      frame "Chien-Hrones-Reswick" {
        n500 = call-poly <vilib>:"PID Autotuning Design.vi"("Tuning specifications"="Tuning specifications 12", "Type of Controller"=w1053, "dt (s)"=w1056, "Response signal"=w1059, "Stimulus signal"=w1060) -> ("PID gains"=w1054:T3, "response offset"=w1057:dbl, "stimulus offset"=w1058:dbl, "Plant Parameters"=w1055:T5)  [unwired: 3 in]
      }
      frame "Internal Model Control" {
        n501 = call-poly <vilib>:"PID Autotuning Design.vi"("Desired Time Constant (tau_c)"="Multiplicative factor 12", "Type of Controller"=w1062, "dt (s)"=w1065, "Response signal"=w1068, "Stimulus signal"=w1069) -> ("PID gains"=w1063:T3, "response offset"=w1066:dbl, "stimulus offset"=w1067:dbl, "Plant Parameters"=w1064:T5)  [unwired: 3 in]
      }
    }
    "Identified Plant Parameters 12" <- w1019
    "Response operating point 12" <- w1021
    "Stimulus operating point 12" <- w1020
    n502 = Unbundle(w1024) -> ("proportional gain (Kc)"=w1027:dbl)  [unwired: 2 out]
    n503 = Equal?(x=w1027, y=inf) -> (x = y?=w1026:bool)
    n504 = feedback #16() -> (w1025:T3)  [unwired: 1 in]
    n505 = Select(t=w1025, s=w1026, f=w1024) -> (s? t:f=w1023:T3)
    "Tuned PID gains 12" <- w1023
    n506 = feedback-in #16(w1023) -> ()
    n507 = case shown="True" "Accept gain 12" {
      tunnel: w1023 -> [_ w1070]
      frame False {
      }
      frame True {
        n508 = local write "PID Gains 12"(w1070) -> ()
      }
    }
    n509 = local read "Stop 12"() -> (w1032:bool)
  }
  n510 = while {
    tunnel: w34 -> [_]
    tunnel: w30 -> [w1074]
    stop <- w1084 stop-if-true
    # "If dT and deadtime have similar values, the identification could evaluate deadtime as zero and this generates proportional gain equal to Inf. This code avoid gain changes in this situations."
    # "Autotuning Loop"
    n511 = local read "Control Output 8"() -> (w1086:dbl[])
    n512 = local read "Measurement 8"() -> (w1085:dbl[])
    n513 = case shown="\"Chien-Hrones-Reswick\"" "Control 8" {
      tunnel: w1086 -> [w1095 w1103 w1112 w1121]
      tunnel: w1085 -> [w1094 w1102 w1111 w1120]
      tunnel: [w1093 w1101 w1110 w1119] -> w1073
      tunnel: [w1092 w1100 w1109 w1118] -> w1072
      tunnel: w1074 -> [w1091 w1099 w1108 w1117]
      tunnel: [w1090 w1098 w1107 w1116] -> w1071
      tunnel: [w1089 w1097 w1106 w1115] -> w1076
      tunnel: "Type of controller 8" -> [w1088 w1096 w1105 w1114]
      frame "Ziegler-Nichols", Default {
        n514 = call-poly <vilib>:"PID Autotuning Design.vi"("Ziegler-Nichols Speed"="Ziegler-Nichols speed 8", "Type of Controller"=w1088, "dt (s)"=w1091, "Response signal"=w1094, "Stimulus signal"=w1095) -> ("PID gains"=w1089:T3, "response operating point"=w1092:dbl, "stimulus operating point"=w1093:dbl, "Plant Parameters"=w1090:T5)  [unwired: 3 in]
      }
      frame "Cohen-Coon" {
        n515 = call-poly <vilib>:"PID Autotuning Design.vi"("Type of Controller"=w1096, "dt (s)"=w1099, "Response signal"=w1102, "Stimulus signal"=w1103) -> ("PID gains"=w1097:T3, "response offset"=w1100:dbl, "stimulus offset"=w1101:dbl, "Plant Parameters"=w1098:T5)  [unwired: 4 in]
      }
      frame "Chien-Hrones-Reswick" {
        n516 = call-poly <vilib>:"PID Autotuning Design.vi"("Tuning specifications"="Tuning specifications 8", "Type of Controller"=w1105, "dt (s)"=w1108, "Response signal"=w1111, "Stimulus signal"=w1112) -> ("PID gains"=w1106:T3, "response offset"=w1109:dbl, "stimulus offset"=w1110:dbl, "Plant Parameters"=w1107:T5)  [unwired: 3 in]
      }
      frame "Internal Model Control" {
        n517 = call-poly <vilib>:"PID Autotuning Design.vi"("Desired Time Constant (tau_c)"="Multiplicative factor 8", "Type of Controller"=w1114, "dt (s)"=w1117, "Response signal"=w1120, "Stimulus signal"=w1121) -> ("PID gains"=w1115:T3, "response offset"=w1118:dbl, "stimulus offset"=w1119:dbl, "Plant Parameters"=w1116:T5)  [unwired: 3 in]
      }
    }
    "Stimulus operating point 8" <- w1073
    "Response operating point 8" <- w1072
    "Identified Plant Parameters 8" <- w1071
    n518 = Unbundle(w1076) -> ("proportional gain (Kc)"=w1079:dbl)  [unwired: 2 out]
    n519 = Equal?(x=w1079, y=inf) -> (x = y?=w1078:bool)
    n520 = feedback #17() -> (w1077:T3)  [unwired: 1 in]
    n521 = Select(t=w1077, s=w1078, f=w1076) -> (s? t:f=w1075:T3)
    "Tuned PID gains 8" <- w1075
    n522 = feedback-in #17(w1075) -> ()
    n523 = case shown="True" "Accept gain 8" {
      tunnel: w1075 -> [_ w1122]
      frame False {
      }
      frame True {
        n524 = local write "PID Gains 8"(w1122) -> ()
      }
    }
    n525 = local read "Stop 8"() -> (w1084:bool)
  }
  n526 = while {
    tunnel: w40 -> [_]
    tunnel: w36 -> [w1126]
    stop <- w1136 stop-if-true
    # "If dT and deadtime have similar values, the identification could evaluate deadtime as zero and this generates proportional gain equal to Inf. This code avoid gain changes in this situations."
    # "Autotuning Loop"
    n527 = local read "Control Output 7"() -> (w1138:dbl[])
    n528 = local read "Measurement 7"() -> (w1137:dbl[])
    n529 = case shown="\"Chien-Hrones-Reswick\"" "Control 7" {
      tunnel: w1138 -> [w1147 w1155 w1164 w1173]
      tunnel: w1137 -> [w1146 w1154 w1163 w1172]
      tunnel: [w1145 w1153 w1162 w1171] -> w1125
      tunnel: [w1144 w1152 w1161 w1170] -> w1124
      tunnel: w1126 -> [w1143 w1151 w1160 w1169]
      tunnel: [w1142 w1150 w1159 w1168] -> w1123
      tunnel: [w1141 w1149 w1158 w1167] -> w1128
      tunnel: "Type of controller 7" -> [w1140 w1148 w1157 w1166]
      frame "Ziegler-Nichols", Default {
        n530 = call-poly <vilib>:"PID Autotuning Design.vi"("Ziegler-Nichols Speed"="Ziegler-Nichols speed 7", "Type of Controller"=w1140, "dt (s)"=w1143, "Response signal"=w1146, "Stimulus signal"=w1147) -> ("PID gains"=w1141:T3, "response operating point"=w1144:dbl, "stimulus operating point"=w1145:dbl, "Plant Parameters"=w1142:T5)  [unwired: 3 in]
      }
      frame "Cohen-Coon" {
        n531 = call-poly <vilib>:"PID Autotuning Design.vi"("Type of Controller"=w1148, "dt (s)"=w1151, "Response signal"=w1154, "Stimulus signal"=w1155) -> ("PID gains"=w1149:T3, "response offset"=w1152:dbl, "stimulus offset"=w1153:dbl, "Plant Parameters"=w1150:T5)  [unwired: 4 in]
      }
      frame "Chien-Hrones-Reswick" {
        n532 = call-poly <vilib>:"PID Autotuning Design.vi"("Tuning specifications"="Tuning specifications 7", "Type of Controller"=w1157, "dt (s)"=w1160, "Response signal"=w1163, "Stimulus signal"=w1164) -> ("PID gains"=w1158:T3, "response offset"=w1161:dbl, "stimulus offset"=w1162:dbl, "Plant Parameters"=w1159:T5)  [unwired: 3 in]
      }
      frame "Internal Model Control" {
        n533 = call-poly <vilib>:"PID Autotuning Design.vi"("Desired Time Constant (tau_c)"="Multiplicative factor 7", "Type of Controller"=w1166, "dt (s)"=w1169, "Response signal"=w1172, "Stimulus signal"=w1173) -> ("PID gains"=w1167:T3, "response offset"=w1170:dbl, "stimulus offset"=w1171:dbl, "Plant Parameters"=w1168:T5)  [unwired: 3 in]
      }
    }
    "Stimulus operating point 7" <- w1125
    "Response operating point 7" <- w1124
    "Identified Plant Parameters 7" <- w1123
    n534 = Unbundle(w1128) -> ("proportional gain (Kc)"=w1131:dbl)  [unwired: 2 out]
    n535 = Equal?(x=w1131, y=inf) -> (x = y?=w1130:bool)
    n536 = feedback #18() -> (w1129:T3)  [unwired: 1 in]
    n537 = Select(t=w1129, s=w1130, f=w1128) -> (s? t:f=w1127:T3)
    "Tuned PID gains 7" <- w1127
    n538 = feedback-in #18(w1127) -> ()
    n539 = case shown="True" "Accept gain 7" {
      tunnel: w1127 -> [_ w1174]
      frame False {
      }
      frame True {
        n540 = local write "PID Gains 7"(w1174) -> ()
      }
    }
    n541 = local read "Stop 7"() -> (w1136:bool)
  }
  n542 = call <instrlib>:"PDI close.vi"("error in (no error)"=w65, "pDev"=w71) -> ("error out"=→"error out":errorcluster, "connected"=w66:bool)  [unwired: 8 out]
  n543 = local write "Connected"(w66) -> ()
